vi "Jarvis.vi"() -> ()   [LabVIEW 2019]
uses:
  <vilib>/Utility/miscctls.llb/LVRectTypeDef.ctl
  controls/GlobalExp.vi
  Global.lvlib
  controls/MasterExpControl.ctl
  VIs/Log/GlobalPyConsole.vi
  <vilib>/rvi/interface/nirviOpenFPGA/nirviOpenFPGA.xnode
  <vilib>/rvi/interface/nirviMethod/nirviMethod.xnode
  VIs/GlobalImagingStatus.vi
  controls/ImagingStatusControl.ctl
  controls/xVerticalSlide/XVerticalSlide.xctl
  controls/xHorizontalSlide/XHorizontalSlide.xctl
  VIs/DataFile/DataLock.vi
  VIs/Graphs/GraphsQueue.vi
  controls/xAOMSettings/XAOMsetting.xctl
  <vilib>/rvi/interface/nirviReadWriteControl/nirviReadWriteControl.xnode
  NiFpgaLv.dll
  <vilib>/Utility/error.llb/Error Cluster From Error Code.vi
  <vilib>/rvi/interface/Simulation/niFpgaSimulationCallBeginRW.vi
  <vilib>/rvi/errors/niLvFpgaAdjustHostInterfaceError.vi
  <vilib>/rvi/interface/nirviCloseFPGA/nirviCloseFPGA.xnode
  VIs/Camera/GlobalCamSettings.vi
  controls/AgilentCtrlEnum.ctl
  FPGA_bitfile/Jarvis_FPGATargetMacro_281119TDCLV2017_HUsPPJBlkv4.lvbitx
  <vilib>/FPGAPlugInAG/Dynamic/niLvFpga_ConfigureFifo_Dynamic.vi
  <vilib>/rvi/errors/niLvFpgaMergeErrorWithErrorCode.vi
  <vilib>/FPGAPlugInAG/Dynamic/niLvFpga_Close_Dynamic.vi
  <vilib>/Utility/file.llb/Write Delimited Spreadsheet (DBL).vi
  <vilib>/FPGAPlugInAG/Dynamic/niLvFpga_ReadFifo_Dynamic.vi
  <vilib>/Utility/file.llb/Write Delimited Spreadsheet (I64).vi
  <vilib>/FPGAPlugInAG/PXI-7842R/niLvFpga_Open_PXI-7842R.vi
  <vilib>/rvi/interface/common/dynamic/niFpgaDynamicAddResources.vi
  <vilib>/Utility/file.llb/Read Delimited Spreadsheet (DBL).vi
  VIs/Qalibrate/exp_status.vi
  VIs/PulseCompiler/CompilerSettings.ctl
  controls/ConnectionStatus.ctl
  controls/FilePaths.ctl
  VIs/Mathematica/MathematicaSettingsCtl.ctl
  VIs/Meta/QueueControl.ctl
  controls/ReadoutSettings.ctl
  VIs/Camera/CameraCoordsControl.ctl
  controls/xTextCode/XTextCode.xctl
  controls/PltImageControl.ctl
  controls/FluoSettings.ctl
  controls/CompCoilControl.ctl
  VIs/RSNRPZ/RSNRPZcontrol.ctl
  controls/ControllerSettings.ctl
  controls/PowerStableSettings.ctl
  <vilib>/userDefined/High Color/nirio_resource_hc.ctl
  controls/AWGchannelcontrol.ctl
  controls/AWGpulse.ctl
  VIs/Shutters/XControl/XControlShutter.xctl
panel:
  out "output 2":i32
  out "time string":string
  in  "dummy cluster":T1
  in  "935 cluster":T1 {"wavelength" format="%_8g"}
  in  "399 cluster":T1 {"wavelength" format="%_8g"}
  in  "739 cluster":T1 {"wavelength" format="%_8g"}
  in  "MasterTabCtl":T2(tab)
  in  "ExperimentTab":enum32{"Control", "Meta Queue", "Settings"}(tab)
  out "runs slider":dbl(slide) scale=0.0..1.0
  out "ExpNumIndicator":string="Experiment # : 000"
  in  "Main/Meta":bool
  in  "RunExp":bool
  out "ExpLog":string="28/02/19 Experiment Logbook:\n000: Frequency scan plus1\n001: Two ion state detection\nError: Interrupted during run 23, lost probe lock."
  out "steps slider":dbl(slide) scale=0.0..1.0
  in  "Pause/Stop":cluster{"Exp Stop":bool, "Pause":bool}
  in  "QueueControl":T3
  in  "LoadExpLog":bool
  in  "SaveExpLog":bool
  in  "ControllerSettings":T4={"Aux Sequence"=FALSE, "Camera"=FALSE, "Recrystallize"=TRUE, "Raw graph"=TRUE, "Mean graph"=TRUE, "Calculate probs"=TRUE, "Find fit"=TRUE, "ReX Time [s] :"=20.0, "Lock Voltage :"=220.0, "Line trig "=FALSE, "Check Fluo"=FALSE, "Pre Sequence"=FALSE}
  out "Aux graph":cluster{dbl, dbl}(graph)
  out "Raw graph":dbl[][](graph)
  out "Mean graph":dbl[][](graph)
  out "Proc. graph":dbl[][](graph)
  out "PltPic":picture
  in  "MathImageCtl":T5={"Date:"="", "Exp Num:"="", "Reload"=FALSE, "Auto update : "=TRUE, "String"=""}
  out "String 3":string="Meta  :"
  in  "MetaPush":bool
  in  "MetaSave":bool
  in  "MetaLoad":bool
  out "Python Console":string
  in  "Param Cfg Path":path=path "C:/Users/cv222/Documents/Jarvis/config/parameter_config.ini"
  in  "Param Cfg add":bool
  in  "Param Cfg Save":bool
  in  "Param Cfg Load":bool
  in  "ConfigHeader":string(combo)
  out "String 2":string="Aux  :"
  out "String":string="Main : "
  in  "AuxCompile":bool
  in  "AuxSave":bool
  in  "AuxLoad":bool
  in  "MainCompile":bool
  in  "MainSave":bool
  in  "MainLoad":bool
  in  "ScriptsTab":T6(tab)
  in  "MainPulsecode":string(xcontrol)
  in  "AuxPulseCode":string(xcontrol)
  in  "MetaPulseCode":string(xcontrol)
  in  "ParamCfgList":string[][](array[string])
  in  "NumIonsProcProbs":bool
  in  "Step Number :":dbl
  in  "AverageCamera":bool
  in  "DisplayImage":bool
  in  "InfoTxtList":string[](array[string])
  in  "Analyze Probs":bool
  in  "Find Probabilites":bool
  in  "Process Statedet":bool
  out "Prob graph":dbl[][](graph)
  out "PostProcImg":picture
  out "Console Out":string
  out "Python Error Out":string
  in  "TreeFolderPath":path=path "C:/Users/labadmin/Documents/Jarvis/data" caption="Base Path"
  in  "DataTree":string(tree)
  out "PostProcCamImg":dbl[][](graph)
  in  "LoadPulseSeq":bool
  in  "Pulse Sequence Tab":T7(tab)
  in  "AuxPulseSeq":T8(array[cluster])
  in  "MainPulseSeq":T8(array[cluster])
  out "RF sequence array":T9[](array[typedef])
  out "MW sequence array":T9[](array[typedef]) {"Channel Array"."phase det" format="%#_10g"; "Channel Array"."amp det" format="%#_10g"; "Channel Array"."freq" format="%#_10g"}
  out "AWGgraph":dbl(graph)
  in  "UpdateAWGSeqGraph":bool
  out "pulseseq parameter config":string
  out "Fluorescence :":dbl
  in  "Shutdown Status :":string
  in  "DisconnectCamera":bool
  in  "CamFluo selector":string(combo)="Large View"
  in  "Large cam coords":T11={"Top :"=450.0, "Bottom :"=280.0, "Left :"=340.0, "Right :"=530.0} caption="Camera Coordinates"
  in  "CamXSlide":cluster{"low":i16, "high":i16}(xcontrol)={"low"=318, "high"=527}
  in  "CamYSlider":cluster{"low":i16, "high":i16}(xcontrol)={"low"=194, "high"=343}
  in  "ion coords":T11={"Top :"=681.0, "Bottom :"=691.0, "Left :"=393.0, "Right :"=406.0}
  out "Big Camera":dbl[][](graph)
  out "CamFluoChart":cluster{"Frequency Chart":u32, "mean":dbl}(graph)
  out "Left ion graph":dbl[][](graph)
  out "Rolling average :":dbl format="%_4g"
  in  "Agilient visa":string="TCPIP0::192.168.1.203::inst0::INSTR" caption="Agilient VSG Resource Name :"
  in  "RSNPRZsettings":T12={"Average Counts :"=1.0, "Correction Freq [MHz] :"=50.0, "Integration Time [ms] : "=0.1, "P :"=0.0, "I :"=0.0, "D :"=0.0, "Power setpoint :"=0.0, "PID on :"=FALSE, "Voltage :"=0.0, "Reset :"=FALSE, "Agilient Power Level [dBm] :"=0.0} caption="RSNPRZ Settings :" {"Agilient Power Level [dBm] :" format="%_4g"; "Voltage :" format="%_5g"; "Power setpoint :" format="%_4g"; "D :" format="%_4g"; "I :" format="%_4g"; "P :" format="%_4g"; "Integration Time [ms] :" format="%_3g"; "Correction Freq [MHz] :" format="%_4g"}
  in  "rsnrpz rsrc name":string="USB::0x0aad::0x00a7::101568" caption="RSNRPZ Resource Name :"
  out "RSNPRZgraph":dbl(graph)
  out "AWGContMSG":string caption="AWG Instrument Response"
  in  "UpdateAWGGraph":bool
  out "Wave Form preview":cluster{"X":dbl, "Y":dbl}[](graph)
  in  "LoadWaveforms":bool
  in  "SaveWaveformsToFile":bool
  in  "SendWaveformToAWG":bool
  in  "Tab Control 2":enum32{"Microwave", "RF"}(tab)
  in  "ArbitraryWaveListTitle":string[][](array[string])=[["Frequency [MHz]", "Amplitude [mV]", "Phase"]] caption="AWGListTitle"
  in  "ArbitraryWaveListMW":dbl[][](array[numeric])=[[100014.0, 200.0, 0.0], [105000.0, 100.0, 0.0], [95000.0, 100.0, 0.0]] caption="Arbitrary Waveform List"
  in  "ArbitraryWaveListRF":dbl[][](array[numeric])=[[100014.0, 200.0, 0.0], [105000.0, 100.0, 0.0], [95000.0, 100.0, 0.0]] caption="Arbitrary Waveform List"
  in  "ArbitraryWaveListTitle 2":string[][](array[string])=[["Frequency [MHz]", "Amplitude [mV]", "Phase"]] caption="AWGListTitle"
  in  "AO cluster":T13
  in  "DIOcluster":T14
  out "AnalogOutput":T15 {"AI 7" scale=0.0..10.0; "AI 6" scale=0.0..10.0; "AI 5" scale=0.0..10.0; "AI 4" scale=0.0..10.0; "AI 3" scale=0.0..10.0; "AI 2" scale=0.0..10.0; "AI 1" scale=0.0..10.0; "AI 0" scale=0.0..10.0}
  in  "369 unlock notification":bool
  in  "VISA: Pressure":refnum<visa-resource-name>
  in  "Tab control":cluster{"visible":bool, "Tab name":string}[](array[cluster])=[{"visible"=TRUE, "Tab name"="Experiment Controller"}, {"visible"=TRUE, "Tab name"="Pulse Programming"}, {"visible"=TRUE, "Tab name"="Pulse Sequence"}, {"visible"=FALSE, "Tab name"="DDS Boards"}, {"visible"=FALSE, "Tab name"="Calypso"}, {"visible"=TRUE, "Tab name"="Digital/Analog"}, {"visible"=FALSE, "Tab name"="Cryo DC"}, {"visible"=FALSE, "Tab name"="Cryo Control"}, {"visible"=TRUE, "Tab name"="Beam Blockers"}]
  in  "LoadSession":bool
  in  "SaveSession":bool
  in  "Mathematica Settings":T16
  in  "Connection Status":T17={"Newton"=TRUE, "Camera"=TRUE, "Atlas"=TRUE, "Pressure"=TRUE, "AWG"=TRUE, "DDS A"=TRUE, "DDS B"=TRUE, "DDS C"=TRUE, "DDS D"=TRUE, "rsnrpz"=TRUE}
  out "GlobalLog":string
  in  "Compiler Settings":T18={"Python Path"=path "", "Main File"="scriptmain.py", "Meta File"="scriptmeta.txt", "Aux File"="scriptaux.py", "Pre File"="scriptpre.py"}
  in  "File Paths":T19={"Local Save Path"=path "C:/Users/cv222/Documents/Jarvis/data", "Newton Save Path"=path "Z:/#Projects/Entanglement/data", "File Name"="test", "LocalSave"=TRUE}
  out "rsnrpz VISA session":refnum<visa-resource-name> caption="VISA resource name"
  in  "FPGA address":T20="PXI1Slot2" caption="RIO Device"
  in  "camera debug":bool
  in  "Stop":bool
  out "Waveform Chart":i32[](graph)
  out "Current iteration":u32
  in  "N measurements":dbl
  in  "Run TDC":bool
  out "FPGAerr":bool=TRUE
  out "Laser status":bool[](array[boolean])
  out "AtlatsStat":string[](array[string])
  in  "Readout Settings":T21={"1ion t'hold (>=)"=3, "2 ion levels?"=FALSE, "2ion t'hold (>=)"=0, "Cam Thresholds"=[4650, 4650], "Region size"=0, "Ion 1 centre x"=3, "Ion 1 centre y"=3, "Ion 2 centre x"=3, "Ion 2 centre y"=3}
  in  "SessionWindowShow":bool
  in  "Global status":enum16{"Idle", "Pulse", "Calypso"}(ring)=enum."Calypso"
  in  "ImagingStatus":enum16{"PMT", "Camera", "Idle"}(ring)=enum."Idle"
  out "Running VIs ref":refnum<vi>[](array[refnum])
  out "queue out":refnum<queue>
  in  "QueueChanged":bool=TRUE
  in  "Stop button":bool
  out "Title":string="Jarvis - IQT Sussex"
  out "Pressure":dbl
  out "Photodiode":dbl
  in  "Small View Tab":enum32{"PMT", "Camera"}(tab)
  out "PMT chart":i32(graph)
  out "Small Camera":dbl[][](graph)
  in  "ExtraTabControl":T22(tab)
  in  "AOMsetting":T23(xcontrol)
  in  "FluoSettings":T24={"Lock Fluorescence"=FALSE, "Aux runs : "=1, "Loop on test :"=FALSE, "Loop frequency : "=FALSE, "Frequency Min"=110.0, "Frequency Max"=130.0, "PMT"={"Lock point : "=68.0, "dF/dFl"=-0.04, "Unlock min"=66.0, "Unlock max"=70.0, "Loop min"=50.0, "Loop max"=160.0}, "Camera"={"Lock point : "=68.0, "dF/dFl"=-0.04, "Unlock min"=66.0, "Unlock max"=70.0, "Loop min"=50.0, "Loop max"=160.0}} {"Camera"."dF/dFl" format="%.2f"; "PMT"."dF/dFl" format="%.2f"}
  in  "CompCoilSettings":T25
  in  "PowerStableSettings":T26={"Lock Power"=TRUE, "Number measurements"=10, "Min AWG Power [dBm] :"=0.0, "Max AWG Power [dBm] :"=1.0, "Min Power Difference [dBm] : "=-1.0, "Max Power Difference [dBm] :"=1.0, "Agilient visa "="TCPIP0::192.168.1.203::inst0::INSTR"}
  in  "XControlShutter":dbl(xcontrol)
  # "Queue :"
  # "AWG trig"
  # "Cam trig"
  # "UWAVE"
  # "countA"
  # "countC"
  # "countD"
  # "countB"
  # "MW5"
  # "AOM"
  # "MW1"
  # "MW2"
  # "MW3"
  # "MW4"
  # "MW6"
  # "MW7"
  # "MW8"
  # "EOM"
  # "DIO9"
  # "trig1"
  # "AO1"
  # "AO2"
  # "AO3"
  # "AO4"
  # "RF1"
  # "RF2"
  # "RF3"
  # "RF5"
  # "RF6"
  # "XM"
  # "RF4"
  # "XR"
  # "Main Sequence"
  # "Auxiliary Sequence"
  # "Name :"
  # "Timing :"
  # "Detuning :"
  # "Step :"
  # "Frequency :"
  # "Step :"
  # "Amplitude :"
  # "Step :"
  # "Phase  :"
  # "Step :"
  # "Name :"
  # "Timing :"
  # "Detuning :"
  # "Step :"
  # "Frequency :"
  # "Step :"
  # "Amplitude :"
  # "Step :"
  # "Phase  :"
  # "Step :"
  # "AOM"
  # "CAM"
  # "MW7"
  # "MW8"
  # "XM"
  # "RF"
  # "XR"
  # "AOM"
  # "EOM"
  # "MW"
  # "MW1"
  # "MW2"
  # "MW3"
  # "MW4"
  # "MW5"
  # "MW6"
  # "Current lock :"
  # "Unlock if :"
  # "Probability lock :"
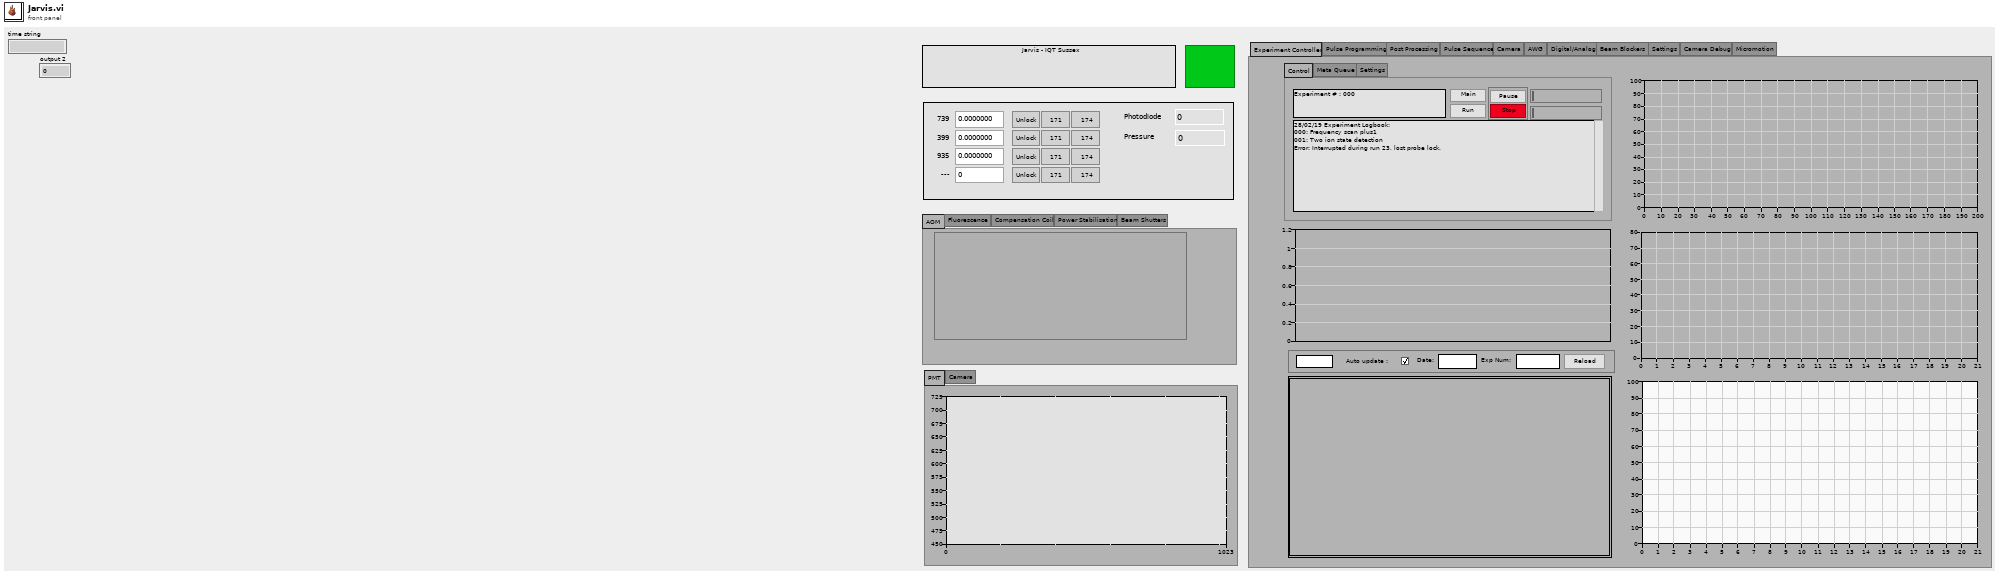
[diagram p1: front panel]
types:
  T1 = cluster{"wavelength":dbl, "unlock":bool, "unlock 2":bool, "unlock 3":bool}
  T2 = enum32{"Experiment Controller", "Pulse Programming", "Post Processing", "Pulse Sequence", "Camera", "AWG", "Calypso", "Digital/Analog", "Beam Blockers", "Cryo Control", "Cryo DC", "Settings", "Camera Debug", "Micromotion", "Debug", "Misc"}
  T3 = typedef "QueueControl.ctl" = cluster{"QueueFromServer":i32, "First Queue":string, "Add To Queue:":string, "Up":bool, "Down":bool, "Del":bool, "Front":bool, "Back":bool, "Next":bool, "Combo Box":string}
  T4 = typedef "ControllerSettings.ctl" = cluster{"Aux Sequence":bool, "Camera":bool, "Recrystallize":bool, "Raw graph":bool, "Mean graph":bool, "Calculate probs":bool, "Find fit":bool, "ReX Time [s] :":dbl, "Lock Voltage :":dbl, "Line trig ":bool, "Check Fluo":bool, "Pre Sequence":bool}
  T5 = typedef "PltImageControl.ctl" = cluster{"Date:":string, "Exp Num:":string, "Reload":bool, "Auto update : ":bool, "String":string}
  T6 = enum32{"Main Script", "Aux Script", "Meta Script"}
  T7 = enum32{"FPGA Sequence", "AWG Sequence", "Parameter Config"}
  T8 = cluster{"String":string, "Numeric":dbl, "Boolean":bool, "Numeric 2":dbl, "Numeric 3":dbl, "Boolean 2":bool, "Boolean 3":bool, "Boolean 4":bool, "Boolean 5":bool, "Boolean 6":bool, "Boolean 7":bool, "Boolean 8":bool, "Boolean 9":bool, "Boolean 10":bool, "Boolean 11":bool, "Boolean 12":bool, "Boolean 13":bool, "Boolean 14":bool, "Boolean 15":bool, "Boolean 16":bool, "Boolean 17":bool, "Boolean 18":bool, "Boolean 19":bool, "Boolean 20":bool, "Boolean 21":bool, "Boolean 22":bool, "Boolean 23":bool, "Boolean 24":bool, "Boolean 25":bool, "Boolean 26":bool, "Boolean 27":bool, "Boolean 28":bool, "Boolean 29":bool, "Boolean 30":bool, "Boolean 31":bool, "Boolean 32":bool, "Boolean 33":bool, "Boolean 34":bool, "Boolean 35":bool, "Boolean 36":bool, "Boolean 37":bool, "Boolean 38":bool, "Boolean 39":bool, "Boolean 40":bool, "Boolean 41":bool, "Boolean 42":bool, "Boolean 43":bool, "Boolean 44":bool, "Boolean 45":bool, "Boolean 46":bool, "Boolean 47":bool, "Boolean 48":bool, "Boolean 49":bool, "Boolean 50":bool, "Boolean 51":bool, "Boolean 52":bool, "Boolean 53":bool, "Boolean 54":bool}[]
  T9 = typedef "AWGpulse.ctl" = cluster{"Name":string, "time det":dbl, "time step":dbl, "Channel Array":T10[]}
  T10 = typedef "AWGchannelcontrol.ctl" = cluster{"freq\n":dbl, "freq step":dbl, "amp det":dbl, "amp step":dbl, "phase det":dbl, "phase step":dbl}
  T11 = typedef "CameraCoordsControl.ctl" = cluster{"Top :":dbl, "Bottom :":dbl, "Left :":dbl, "Right :":dbl}
  T12 = typedef "RSNRPZcontrol.ctl" = cluster{"Average Counts :":dbl, "Correction Freq [MHz] :":dbl, "Integration Time [ms] : ":dbl, "P :":dbl, "I :":dbl, "D :":dbl, "Power setpoint :":dbl, "PID on :":bool, "Voltage :":dbl, "Reset :":bool, "Agilient Power Level [dBm] :":dbl}
  T13 = cluster{"AO 0":dbl, "AO 1":dbl, "AO 2":dbl, "AO 3":dbl, "AO 4":dbl, "AO 5":dbl, "AO 6":dbl, "AO 7":dbl}
  T14 = cluster{"DIO 0":bool, "DIO 1":bool, "DIO 2":bool, "DIO 3":bool, "DIO 4":bool, "DIO 5":bool, "DIO 6":bool, "DIO 7":bool, "DIO 8":bool, "DIO 9":bool, "DIO 10":bool, "DIO 11":bool, "DIO 12":bool, "DIO 13":bool, "DIO 14":bool, "DIO 15":bool, "DIO 16":bool, "DIO 17":bool, "DIO 18":bool, "DIO 19":bool, "DIO 20":bool, "DIO 21":bool, "DIO 22":bool, "DIO 23":bool, "DIO 24":bool, "DIO 25":bool, "DIO 26":bool, "DIO 27":bool, "DIO 28":bool, "DIO 29":bool, "DIO 30":bool, "DIO 31":bool, "DIO 32":bool, "DIO 33":bool, "DIO 34":bool, "DIO 35":bool, "DIO 36":bool, "DIO 37":bool, "DIO 38":bool, "DIO 39":bool}
  T15 = cluster{"AI 0":dbl, "AI 1":dbl, "AI 2":dbl, "AI 3":dbl, "AI 4":dbl, "AI 5":dbl, "AI 6":dbl, "AI 7":dbl}
  T16 = typedef "MathematicaSettingsCtl.ctl" = cluster{"Mathematica Dir":path, "Scripts Dir":path}
  T17 = typedef "ConnectionStatus.ctl" = cluster{"Newton":bool, "Camera":bool, "Atlas":bool, "Pressure":bool, "AWG":bool, "DDS A":bool, "DDS B":bool, "DDS C":bool, "DDS D":bool, "rsnrpz":bool}
  T18 = typedef "CompilerSettings.ctl" = cluster{"Python Path":path, "Main File":string, "Meta File":string, "Aux File":string, "Pre File":string}
  T19 = typedef "FilePaths.ctl" = cluster{"Local Save Path":path, "Newton Save Path":path, "File Name":string, "LocalSave":bool}
  T20 = typedef "nirio_resource_hc.ctl" = tag
  T21 = typedef "ReadoutSettings.ctl" = cluster{"1ion t'hold (>=)":u32, "2 ion levels?":bool, "2ion t'hold (>=)":u32, "Cam Thresholds":u32[], "Region size":i32, "Ion 1 centre x":i32, "Ion 1 centre y":i32, "Ion 2 centre x":i32, "Ion 2 centre y":i32}
  T22 = enum32{"AOM", "Fluorescence", "Compensation Coil", "Power Stabilisation", "Beam Shutters"}
  T23 = cluster{"HighPowerNum":dbl, "LowPowerNum":dbl, "PIDnum":dbl, "DeltaFreq":dbl, "BaseFreq":dbl, "AOMout":dbl, "ButtonSelected":enum16{"PID", "Low", "High"}, "AO3":bool}
  T24 = typedef "FluoSettings.ctl" = cluster{"Lock Fluorescence":bool, "Aux runs : ":i32, "Loop on test :":bool, "Loop frequency : ":bool, "Frequency Min":dbl, "Frequency Max":dbl, "PMT":cluster{"Lock point : ":dbl, "dF/dFl":dbl, "Unlock min":dbl, "Unlock max":dbl, "Loop min":dbl, "Loop max":dbl}, "Camera":cluster{"Lock point : ":dbl, "dF/dFl":dbl, "Unlock min":dbl, "Unlock max":dbl, "Loop min":dbl, "Loop max":dbl}}
  T25 = typedef "CompCoilControl.ctl" = cluster{"Min [mA]":dbl, "Max [mA]":dbl, "Apply lock :":bool, "Unlock min":dbl, "Unlock max":dbl, "Loop current :":bool, "Reset if out of range :":bool, "Aux runs :":i32, "dI [mA] :":dbl, "Prob lock min ":dbl, "Prob lock max":dbl, "Current [mA]":dbl}
  T26 = typedef "PowerStableSettings.ctl" = cluster{"Lock Power":bool, "Number measurements":i32, "Min AWG Power [dBm] :":dbl, "Max AWG Power [dBm] :":dbl, "Min Power Difference [dBm] : ":dbl, "Max Power Difference [dBm] :":dbl, "Agilient visa ":string}
  T27 = typedef "ImagingStatusControl.ctl" = enum16{"PMT_large", "Camera_large", "PMT", "Camera", "Idle"}
  T28 = enum8{"Enabled", "Disabled", "Disabled and Grayed Out"}
  T29 = enum16{"Innit", "Stop", "Idle", "MainRunning", "AuxRunning"}
  T30 = enum32{"Page Enabled", "Page Disabled", "Page Disabled & Grayed"}
  T31 = typedef "MasterExpControl.ctl" = cluster{"Main Steps":dbl, "Main Runs":dbl, "ExpStatus":enum16{"Innit", "Stop", "Idle", "MainRunning", "AuxRunning"}, "Main Current Step":dbl, "ExpNum":dbl, "NewData":bool, "date":string, "command":string, "Stop":bool, "Pause":bool, "Mathematica":string, "Main/Meta":bool, "UpdateMath":bool, "Camera":bool, "MetaExpOver":bool, "NextMetaExp":bool}
  T32 = typedef "LVRectTypeDef.ctl" = cluster{"Left":i16, "Top":i16, "Right":i16, "Bottom":i16}
  T33 = enum16{"del", "update", "down", "up", "bot", "top"}
  T34 = typedef "AgilentCtrlEnum.ctl" = enum16{"WRITE_POW", "READ_POW"}
  T35 = cluster{"Wavelengths[0]":dbl, "Wavelengths[1]":dbl, "Wavelengths[2]":dbl, "Wavelengths[3]":dbl, "Wavelengths[4]":dbl, "Wavelengths[5]":dbl, "Wavelengths[6]":dbl, "Wavelengths[7]":dbl, "Wavelengths[8]":dbl}
  T36 = typedef "SinglePulse.ctl" = cluster{"enabled":bool, "string":string, "time":dbl, "step":dbl, "dio":dbl, "count":dbl, "trigger":dbl, "AO":dbl}
  T37 = cluster{"Pulse name":string, "Pulse number":i32, "Enabled?":bool, "Time":dbl, "Step":dbl, "Pulse 0":bool, "Pulse 1":bool, "Pulse 2":bool, "Pulse 3":bool, "Pulse 4":bool, "Pulse 5":bool, "Pulse 6":bool, "Pulse 7":bool, "Pulse 8":bool, "Pulse 9":bool, "Pulse 10":bool, "Pulse 11":bool, "Pulse 12":bool, "Pulse 13":bool, "Pulse 14":bool, "Pulse 15":bool, "Pulse 16":bool, "Pulse 17":bool, "Pulse 18":bool, "Pulse 19":bool, "Pulse 20":bool, "Pulse 21":bool, "Pulse 22":bool, "Pulse 23":bool, "Pulse 24":bool, "Pulse 25":bool, "Pulse 26":bool, "Pulse 27":bool, "Pulse 28":bool, "Pulse 29":bool, "Pulse 30":bool, "Pulse 31":bool, "Pulse 32":bool, "Pulse 33":bool, "Pulse 34":bool, "Pulse 35":bool, "Pulse 36":bool, "Pulse 37":bool, "Pulse 38":bool, "Pulse 39":bool, "Count 0":bool, "Count 1":bool, "Count 2":bool, "Count 3":bool, "Count 4":bool, "Count 5":bool, "Count 6":bool, "Count 7":bool, "AO 0":bool, "AO 1":bool, "AO 2":bool, "AO 3":bool, "Trigger 0":bool}[]
  T38 = typedef "CameraSettings.ctl" = cluster{"EM Gain :":dbl, "Pre Amp Gain :":dbl, "VS Speed [Index] :":dbl, "VS Amplitude :":dbl, "Exposure Time [s] :":dbl, "Temperature :":dbl, "HS Speed [s]":dbl, "Gain > 300 :":bool}
  T39 = cluster{"number: 0 to 1":dbl, "number: 0 to 1":dbl}
  T40 = cluster{"steps slider":refnum<vi>, "runs slider":refnum<vi>}
  T41 = cluster{"CompCoilSettings":refnum<vi>, "FluoSettings":refnum<vi>, "AOMsetting":refnum<vi>, "PowerStableSettings":refnum<vi>}
  T42 = cluster{"StepsSlider":refnum<vi>, "runs slider":refnum<vi>}
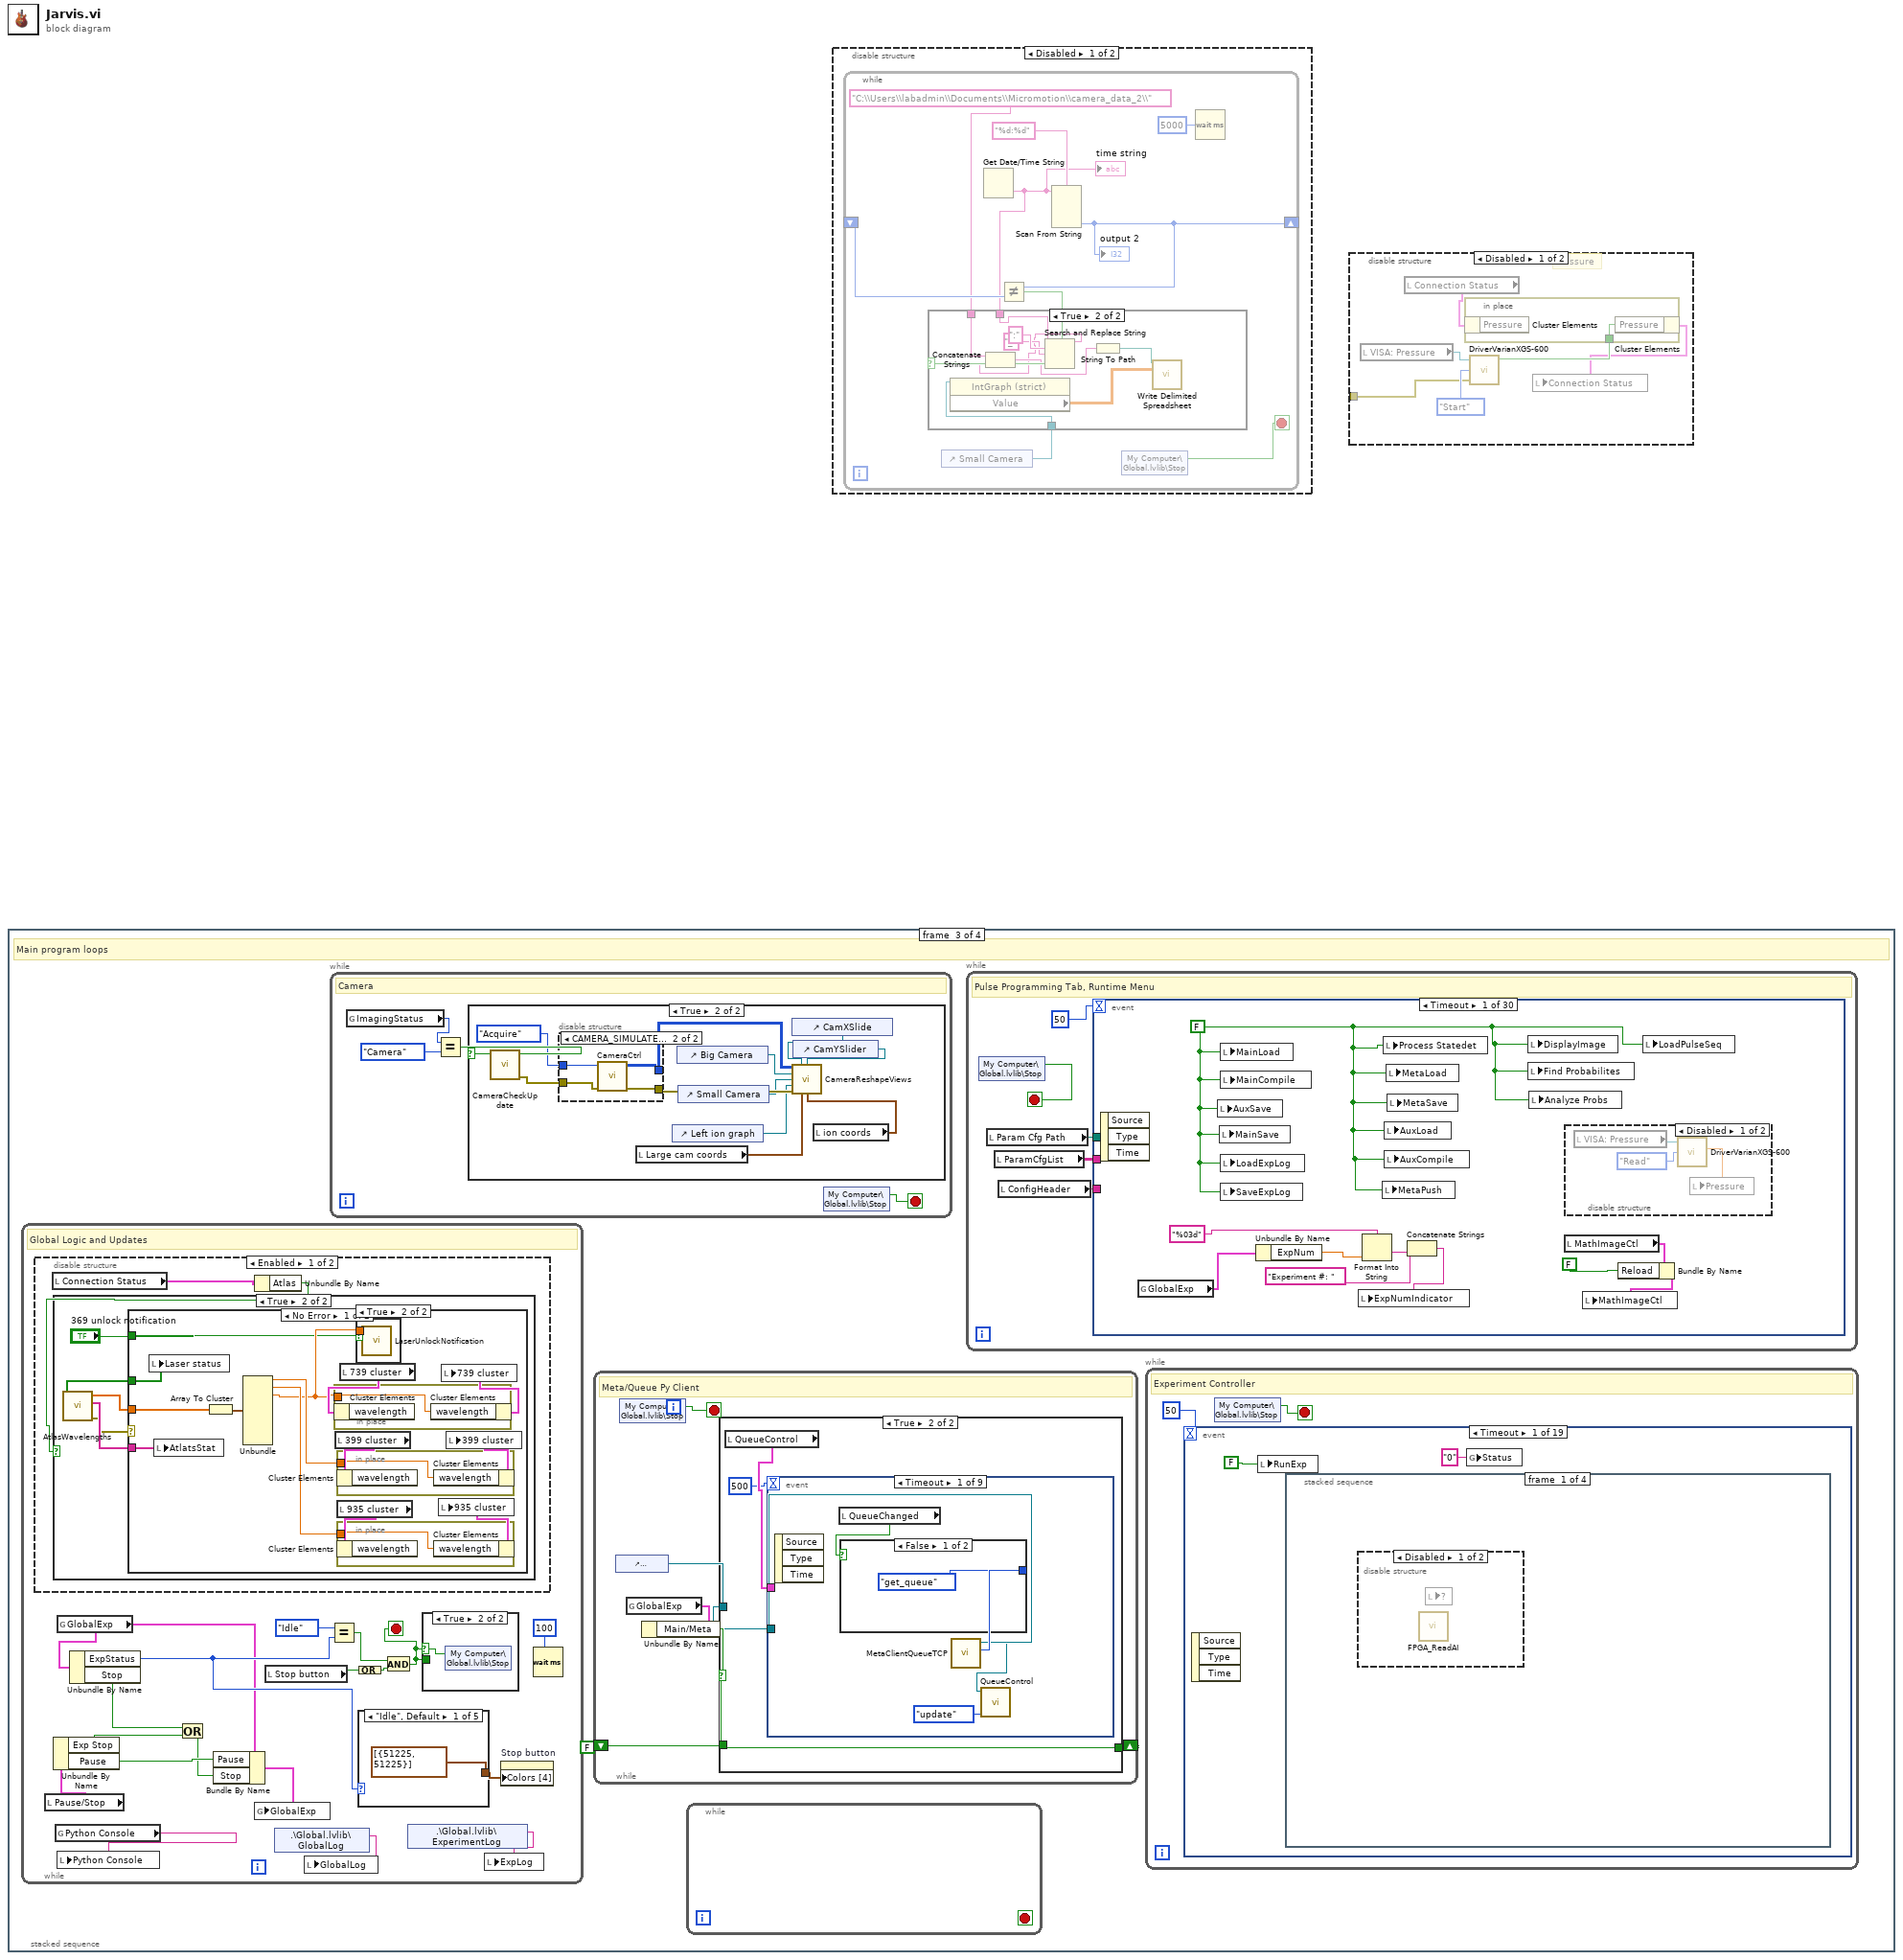
[diagram p0: block diagram]
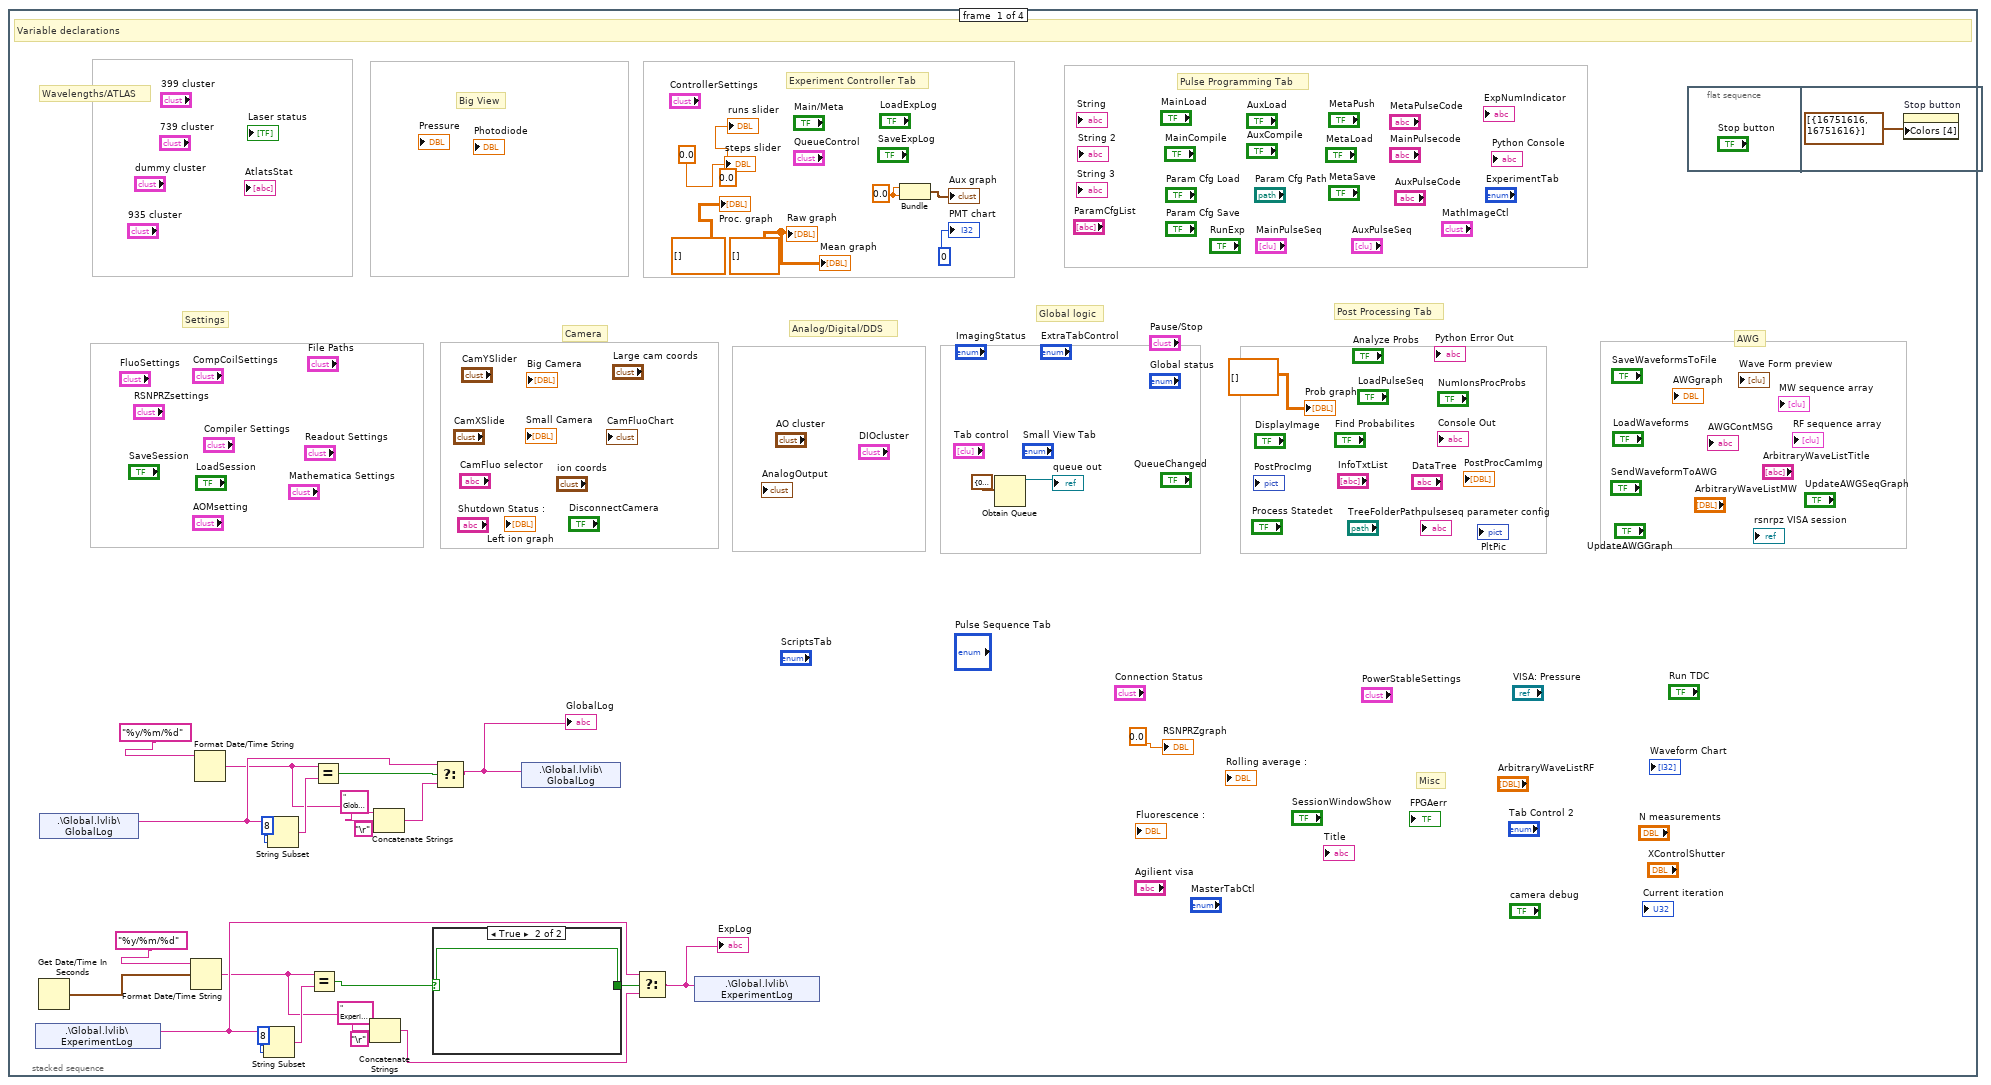
[diagram p5: hidden frame]
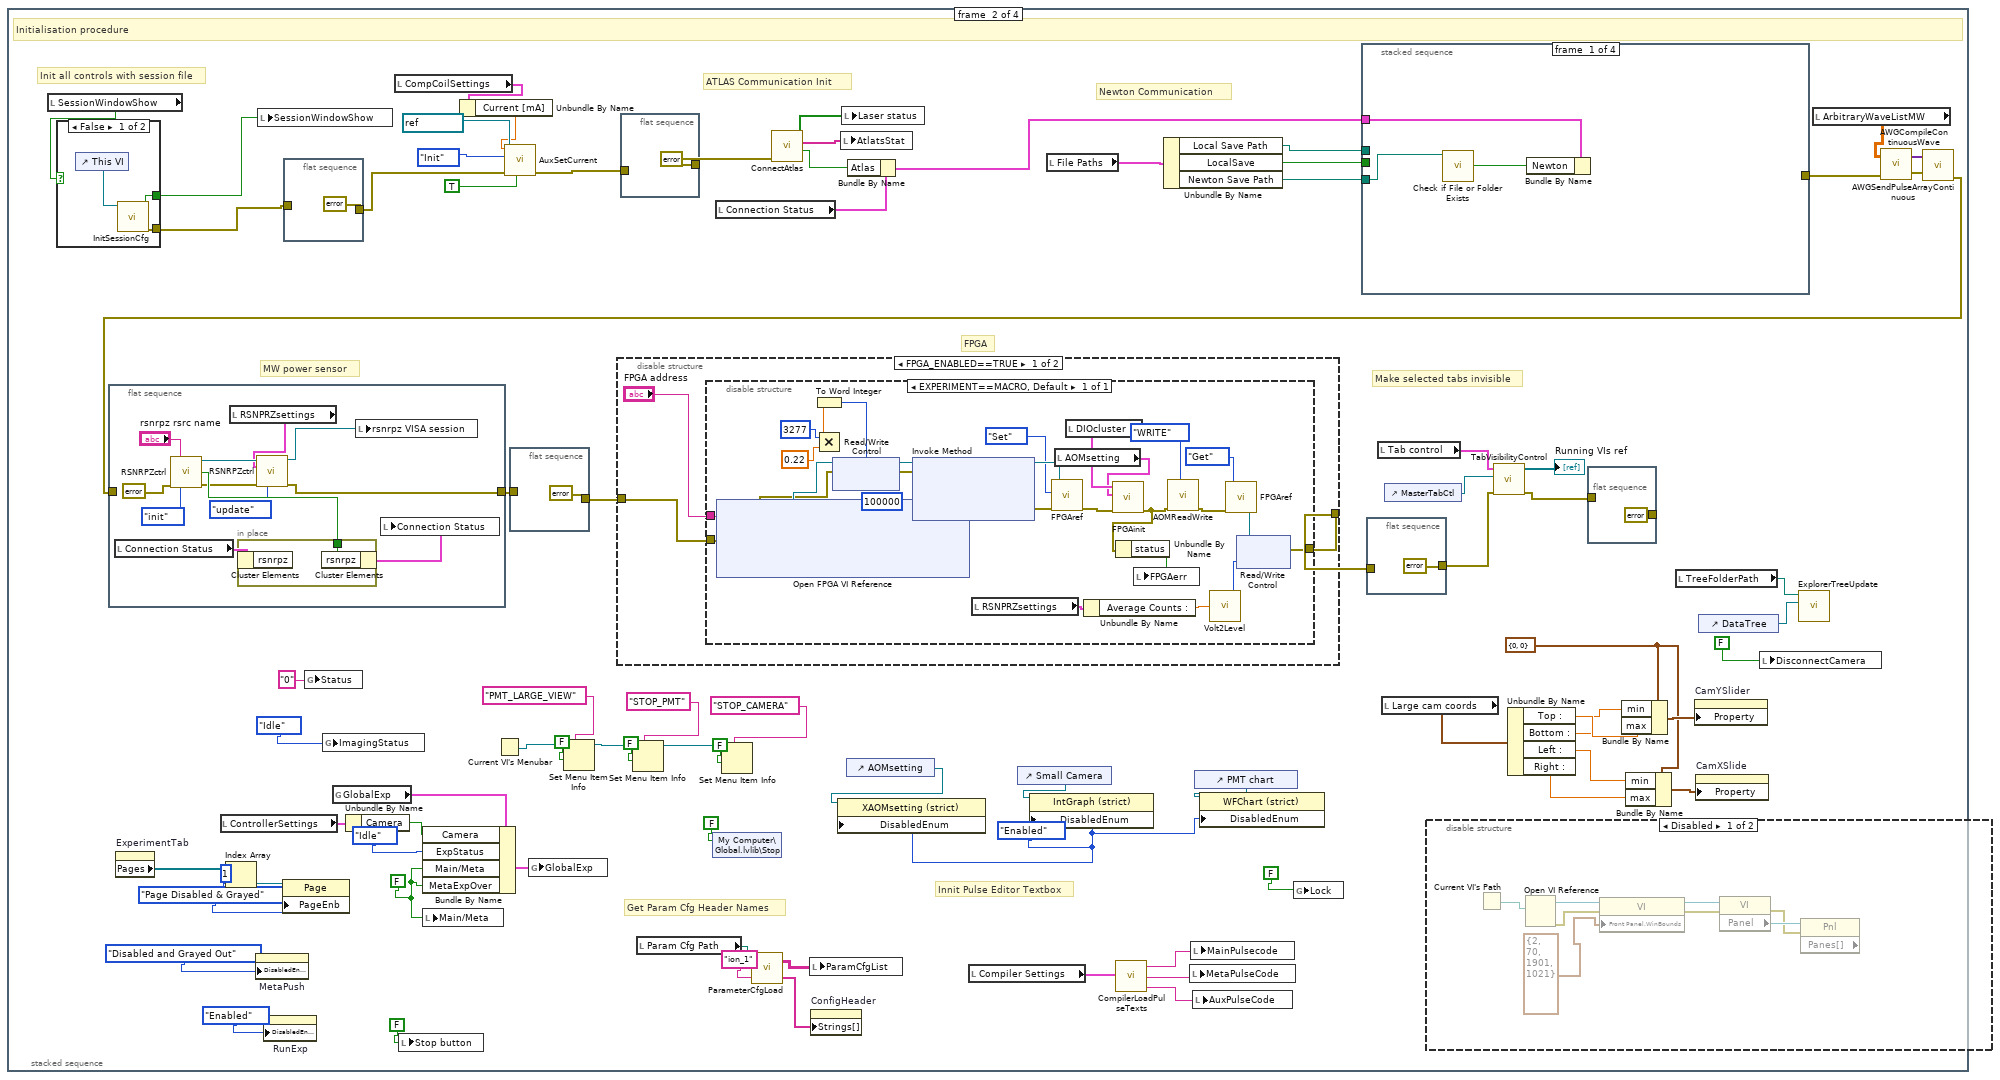
[diagram p7: hidden frame]
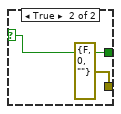
[diagram p9: hidden frame]
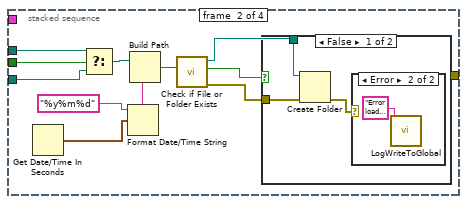
[diagram p10: hidden frame]
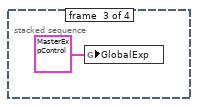
[diagram p13: hidden frame]
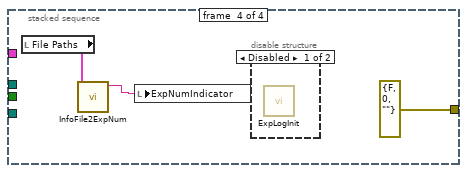
[diagram p14: hidden frame]
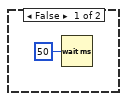
[diagram p17: hidden frame]
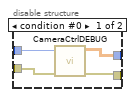
[diagram p18: hidden frame]
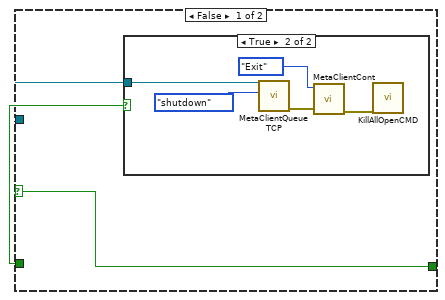
[diagram p19: hidden frame]
diagram:
  n1 = stacked-sequence {
    frame #0 {
      w5 = 0.0
      w23 = dbl[][] []
      # "AWG"
      # "Misc"
      # "Post Processing Tab"
      # "Global logic"
      # "Analog/Digital/DDS"
      # "Settings"
      # "Camera"
      # "Big View"
      # "Experiment Controller Tab"
      # "Pulse Programming Tab"
      # "Wavelengths/ATLAS"
      # "Variable declarations"
      n2 = shared-variable ".\\Global.lvlib\\ExperimentLog"() -> (w30:string)  [unwired: 1 in, 1 out]
      n3 = Get Date/Time In Seconds() -> (seconds since 1Jan1904=w31:timestamp)
      n4 = shared-variable ".\\Global.lvlib\\GlobalLog"() -> (w20:string)  [unwired: 1 in, 1 out]
      n5 = Format Date/Time String(time format string (%c)="%y/%m/%d", seconds (now)=w31) -> (date/time string=w24:string)  [unwired: 1 in]
      n6 = Format Date/Time String(time format string (%c)="%y/%m/%d") -> (date/time string=w15:string)  [unwired: 2 in]
      n7 = String Subset(string=w30, length (rest)=8 ("length (rest)")) -> (substring=w26:string)  [unwired: 1 in]
      n8 = String Subset(string=w20, length (rest)=8 ("length (rest)")) -> (substring=w16:string)  [unwired: 1 in]
      n9 = Equal?(x=w24, y=w26) -> (x = y?=w13:bool)
      n10 = Equal?(x=w15, y=w16) -> (x = y?=w14:bool)
      n11 = Concatenate Strings(w24, " Experiment Logbook:" ("string"), "\r") -> (w27:string)
      n12 = Concatenate Strings(w15, " Global Log:" ("string"), "\r") -> (w17:string)
      n13 = case shown="True" w13 {
        selector: w13 -> [w35 w36]
        tunnel: [w35 w36] -> w12
        frame False {
        }
        frame True {
        }
      }
      n14 = Select(t=w20, s=w14, f=w17) -> (s? t:f=w11:string)
      "GlobalLog" <- w11
      n15 = shared-variable ".\\Global.lvlib\\GlobalLog"(w11) -> ()  [unwired: 1 in, 1 out]
      n16 = Select(t=w30, s=w12, f=w27) -> (s? t:f=w25:string)
      "ExpLog" <- w25
      n17 = shared-variable ".\\Global.lvlib\\ExperimentLog"(w25) -> ()  [unwired: 1 in, 1 out]
      n18 = Bundle(w5, w5) -> (→"Aux graph":cluster{dbl, dbl})  [unwired: 1 in]
      n19 = Obtain Queue(element data type=cluster{dbl, dbl} {0.0, 0.0}) -> (queue out=→"queue out":refnum<queue>)  [unwired: 4 in, 2 out]
      n20 = flat-sequence {
        frame #0 {
        }
        frame #1 {
          n21 = property on="Stop button" class="Bool (strict)"("Colors [4]"=cluster{u32, u32}[] [{16751616, 16751616}]) -> ()  [unwired: 2 in, 2 out]
        }
      }
      "Proc. graph" <- dbl[][] []
      "Mean graph" <- w23
      "Raw graph" <- w23
      "runs slider" <- 0.0 ("runs slider")
      "steps slider" <- 0.0 ("steps slider")
      "PMT chart" <- 0
      "Prob graph" <- dbl[][] []
      "RSNPRZgraph" <- 0.0
    }
    frame #1 {
      w77 = cluster{"min":i16, "max":i16} {"min"=0, "max"=0} ("SlideBounds")
      w60 = T28."Enabled" ("Disabled")
      w51 = FALSE ("Main/Meta")
      # "MW power sensor"
      # "FPGA"
      # "Init all controls with session file"
      # "Make selected tabs invisible"
      # "Innit Pulse Editor Textbox"
      # "Get Param Cfg Header Names"
      # "Newton Communication"
      # "ATLAS Communication Init"
      # "Initialisation procedure"
      n22 = local read "SessionWindowShow"() -> (w99:bool)
      n23 = case shown="False" w99 {
        selector: w99 -> [_ w172]
        tunnel: [w171 errorcluster {"status"=FALSE, "code"=0, "source"=""} ("error out")] -> w48
        tunnel: [w169 w172] -> w98
        frame False {
          n24 = control-ref of="This VI"() -> (w170:refnum<vi>)
          n25 = call "InitSessionCfg.vi"("This VI"=w170) -> ("error out"=w171:errorcluster, "Showagian 2"=w169:bool)  [unwired: 9 in]
        }
        frame True {
        }
      }
      n26 = flat-sequence {
        tunnel: w52 -> [_]
        tunnel: [w159] -> w59
        frame #0 {
          n27 = local read "Connection Status"() -> (w165:T17)
          n28 = call "RSNRPZctrl.vi"("Resource Name (USB::0x0aad::0x000b::100000)"="rsnrpz rsrc name", "error in (no error)"=errorcluster {"status"=FALSE, "code"=0, "source"=""}, "action"=enum16{"close", "update", "read", "init"}."init") -> ("dup VISA session out"=w162:refnum<visa-resource-name>, "connection status"=w164:bool, "error out"=w161:errorcluster)  [unwired: 9 in, 1 out]
          n29 = local read "RSNPRZsettings"() -> (w156:T12)
          n30 = in-place {
            in-place-border: w164 -> [w168]
            n31 = in-place-cluster #1(w165) -> ()  [unwired: 1 out]
            n32 = in-place-cluster #1("rsnrpz"=w168) -> (w163:T17)
          }
          n33 = call "RSNRPZctrl.vi"("VISA session in"=w162, "RSNPRZsettings"=w156, "error in (no error)"=w161, "action"=enum16{"close", "update", "read", "init"}."update") -> ("dup VISA session out"=w160:refnum<visa-resource-name>, "error out"=w159:errorcluster)  [unwired: 8 in, 2 out]
          n34 = local write "rsnrpz VISA session"(w160) -> ()
          n35 = local write "Connection Status"(w163) -> ()
        }
      }
      n36 = property on="ExperimentTab" class="TabCtl (strict)"() -> ("Pages"=w104:refnum<vi>[])  [unwired: 2 in, 2 out]
      n37 = local read "ControllerSettings"() -> (w68:T4)
      n38 = Index Array(array=w104, index=1) -> (element=w103:refnum<vi>)
      n39 = property on="MetaPush" class="Bool (strict)"("DisabledEnum"=T28."Disabled and Grayed Out" ("Disabled")) -> ()  [unwired: 2 in, 2 out]
      n40 = local write "SessionWindowShow"(w98) -> ()
      n41 = property on="RunExp" class="Bool (strict)"("DisabledEnum"=T28."Enabled" ("Disabled")) -> ()  [unwired: 2 in, 2 out]
      n42 = property class="Page"(reference=w103, "PageEnb"=T30."Page Disabled & Grayed" ("Page Enabled State")) -> ()  [unwired: 1 in, 2 out]
      n43 = flat-sequence {
        tunnel: [errorcluster {"status"=FALSE, "code"=0, "source"=""} ("error out")] -> w47
        tunnel: w48 -> [_]
        frame #0 {
        }
      }
      n44 = global write "exp_status.vi" "Status"("0" ("Status")) -> ()
      n45 = global write "GlobalImagingStatus.vi" "ImagingStatus"(ImagingStatusControl."Idle" ("ImagingStatus")) -> ()
      n46 = global read "GlobalExp.vi" "GlobalExp"() -> (w108:T31)
      n47 = Unbundle By Name(w68) -> ("Camera"=w67:bool)
      n48 = local read "CompCoilSettings"() -> (w42:T25)
      n49 = local write "Stop button"(FALSE ("Stop button")) -> ()
      n50 = Bundle By Name(cluster=w108, "Camera"=w67, "ExpStatus"=T29."Idle", "Main/Meta"=w51, "MetaExpOver"=w51) -> (w107:T31)
      n51 = local write "Main/Meta"(w51) -> ()
      n52 = Unbundle By Name(w42) -> ("Current [mA]"=w41:dbl)
      n53 = Current VI's Menubar() -> (w87:refnum<k9>)
      n54 = call "AuxSetCurrent.vi"("Enabled?"=TRUE, "error in"=w47, "VISA resource name"=refnum<visa-resource-name> "COM8", "Function select"=enum16{"Init", "Set", "Close"}."Init", "current /mA"=w41) -> ("error out"=w46:errorcluster)  [unwired: 4 in, 2 out]
      n55 = flat-sequence {
        tunnel: [errorcluster {"status"=FALSE, "code"=0, "source"=""} ("error out")] -> w63
        tunnel: w59 -> [_]
        frame #0 {
        }
      }
      n56 = global write "GlobalExp.vi" "GlobalExp"(w107) -> ()
      n57 = Set Menu Item Info(7:"PMT_LARGE_VIEW" ("item tag"), 9:FALSE ("enabled"), 11:w87) -> (3:w82:refnum<k9>)  [unwired: 4 in, 1 out]
      n58 = disable-structure shown="FPGA_ENABLED==TRUE" {
        disable-tunnel: w63 -> [w124 w153]
        disable-tunnel: [w123 w153] -> w62
        frame condition #0 (active) {
          n59 = disable-structure shown="EXPERIMENT==MACRO, Default" {
            disable-tunnel: w124 -> [w152]
            disable-tunnel: [w129] -> w123
            disable-tunnel: "FPGA address" -> [w125]
            frame condition #0 (active) {
              n60 = xnode "Open FPGA VI Reference"("error in"=w152, "resource name"=w125) -> ("FPGA VI Reference Out"=w144:refnum<k20>, "error out"=w142:errorcluster)
              n61 = Multiply(x=3277, y=0.22) -> (x*y=w138:dbl)
              n62 = To Word Integer(number=w138) -> (16bit integer=w137:i16)
              n63 = xnode "Read/Write Control"("FPGA VI Reference In"=w144, "error in"=w142, "AO4 max"=w137) -> ("FPGA VI Reference Out"=w143:refnum<k20>, "error out"=w141:errorcluster)
              n64 = xnode "Invoke Method"("FPGA VI Reference In"=w143, "error in"=w141, "Requested Depth"=u32 100000) -> ("FPGA VI Reference Out"=w149:refnum<k20>, "error out"=w150:errorcluster)  [unwired: 1 out]
              n65 = local read "RSNPRZsettings"() -> (w128:T12)
              n66 = call "FPGAref.vi"("error in"=w150, "Enum"=enum16{"Set", "Get"}."Set", "FPGA VI Reference Out"=w149) -> ("error out"=w147:errorcluster)  [unwired: 3 in, 1 out]
              n67 = local read "AOMsetting"() -> (w136:T23)
              n68 = local read "DIOcluster"() -> (w145:T14)
              n69 = Unbundle By Name(w128) -> ("Average Counts :"=w127:dbl)
              n70 = call "FPGAinit.vi"("error in"=w147, "XAOMsetting"=w136, "DIOcluster"=w145) -> ("error out"=w134:errorcluster)  [unwired: 8 in]
              n71 = Unbundle By Name(w134) -> ("status"=w146:bool)
              n72 = local write "FPGAerr"(w146) -> ()
              n73 = call "AOMReadWrite.vi"("Enum"=enum16{"READ", "WRITE"}."WRITE", "error in"=w134) -> ("error out"=w133:errorcluster)  [unwired: 7 in, 2 out]
              n74 = call "Volt2Level.vi"("voltage /V"=w127) -> ("level"=w126:i16)
              n75 = call "FPGAref.vi"("error in"=w133, "Enum"=enum16{"Set", "Get"}."Get") -> ("error out"=w130:errorcluster, "FPGA VI Reference Out 2"=w131:refnum<k20>)  [unwired: 4 in]
              n76 = xnode "Read/Write Control"("FPGA VI Reference In"=w131, "error in"=w130, "AO5"=w126) -> ("error out"=w129:errorcluster)  [unwired: 1 out]
            }
          }
        }
        frame condition #1 {
        }
      }
      n77 = flat-sequence {
        tunnel: [errorcluster {"status"=FALSE, "code"=0, "source"=""} ("error out")] -> w49
        tunnel: w46 -> [_]
        frame #0 {
        }
      }
      n78 = Set Menu Item Info(7:"STOP_PMT" ("item tag"), 9:FALSE ("enabled"), 11:w82) -> (3:w81:refnum<k9>)  [unwired: 4 in, 1 out]
      n79 = local read "Param Cfg Path"() -> (w116:path)
      n80 = shared-variable "My Computer\\Global.lvlib\\Stop"(FALSE ("Stop")) -> ()  [unwired: 1 in, 1 out]
      n81 = local read "Connection Status"() -> (w50:T17)
      n82 = Set Menu Item Info(7:"STOP_CAMERA" ("item tag"), 9:FALSE ("enabled"), 11:w81) -> ()  [unwired: 4 in, 2 out]
      n83 = call "ParameterCfgLoad.vi"("Section"="ion_1", "configuration file path"=w116) -> ("section names list"=w115:string[], "Array - String"=w117:string[][])
      n84 = call "ConnectAtlas.vi"("error in (no error)"=w49) -> ("Atlas connection"=w38:bool, "AtlatsStat"=w39:string[], "Laser status"=w40:bool[])  [unwired: 8 in]
      n85 = local write "ParamCfgList"(w117) -> ()
      n86 = property on="ConfigHeader" class="CmbBox"("Strings[]"=w115) -> ()  [unwired: 2 in, 2 out]
      n87 = local write "AtlatsStat"(w39) -> ()
      n88 = local write "Laser status"(w40) -> ()
      n89 = control-ref of="AOMsetting"() -> (w61:refnum<vi>)
      n90 = property class="XAOMsetting (strict)"(reference=w61, "DisabledEnum"=w60) -> ()  [unwired: 1 in, 2 out]
      n91 = Bundle By Name(cluster=w50, "Atlas"=w38) -> (w109:T17)
      n92 = local read "Compiler Settings"() -> (w71:T18)
      n93 = control-ref of="Small Camera"() -> (w91:refnum<vi>)
      n94 = property class="IntGraph (strict)"(reference=w91, "DisabledEnum"=w60) -> ()  [unwired: 1 in, 2 out]
      n95 = local read "File Paths"() -> (w113:T19)
      n96 = call "CompilerLoadPulseTexts.vi"("compile settings"=w71) -> ("AuxCode 2"=w69:string, "MetaCode 2"=w70:string, "Maincode 2"=w72:string)  [unwired: 2 in]
      n97 = Unbundle By Name(w113) -> ("Local Save Path"=w112:path, "LocalSave"=w111:bool, "Newton Save Path"=w110:path)
      n98 = local write "MetaPulseCode"(w70) -> ()
      n99 = local write "MainPulsecode"(w72) -> ()
      n100 = local write "AuxPulseCode"(w69) -> ()
      n101 = control-ref of="PMT chart"() -> (w92:refnum<vi>)
      n102 = property class="WFChart (strict)"(reference=w92, "DisabledEnum"=w60) -> ()  [unwired: 1 in, 2 out]
      n103 = global write "DataLock.vi" "Lock"(FALSE ("Lock")) -> ()
      n104 = stacked-sequence {
        tunnel: w112 -> [_ w179 _ _]
        tunnel: w111 -> [_ w178 _ _]
        tunnel: w110 -> [w176 w177 _ _]
        tunnel: w109 -> [w174 _ _ _]
        tunnel: [_ _ _ errorcluster {"status"=FALSE, "code"=0, "source"=""} ("error constant")] -> w54
        frame #0 {
          n105 = call <vilib>:"Check if File or Folder Exists.vi"("path"=w176) -> ("file or folder exists?"=w175:bool)  [unwired: 8 in, 2 out]
          n106 = Bundle By Name(cluster=w174, "Newton"=w175) -> ()  [unwired: 1 out]
        }
        frame #1 {
          n107 = Get Date/Time In Seconds() -> (seconds since 1Jan1904=w186:timestamp)
          n108 = Select(t=w179, s=w178, f=w177) -> (s? t:f=w185:path)
          n109 = Format Date/Time String(time format string (%c)="%y%m%d", seconds (now)=w186) -> (date/time string=w184:string)  [unwired: 1 in]
          n110 = Build Path(base path=w185, name or relative path=w184) -> (appended path=w183:path)
          n111 = call <vilib>:"Check if File or Folder Exists.vi"("path"=w183) -> ("error out"=w181:errorcluster, "file or folder exists?"=w182:bool, "dup path"=w180:path)  [unwired: 8 in]
          n112 = case shown="False" w182 {
            tunnel: w181 -> [w190 _]
            tunnel: w180 -> [w189 _]
            frame False {
              n113 = Create Folder(path (use dialog)=w189, error in=w190) -> (error out=w188:errorcluster)  [unwired: 1 in, 2 out]
              n114 = case shown="Error" w188 {
                frame No Error {
                }
                frame Error {
                  n115 = call "LogWriteToGlobal.vi"("in string"="Error loading/creating data folder: invalid path.") -> ()  [unwired: 11 in]
                }
              }
            }
            frame True {
            }
          }
        }
        frame #2 {
          n116 = global write "GlobalExp.vi" "GlobalExp"(T31 {"Main Steps"=0.0, "Main Runs"=0.0, "ExpStatus"=enum."Idle", "Main Current Step"=0.0, "ExpNum"=0.0, "NewData"=FALSE, "date"="", "command"="", "Stop"=FALSE, "Pause"=FALSE, "Mathematica"="", "Main/Meta"=FALSE, "UpdateMath"=FALSE, "Camera"=FALSE, "MetaExpOver"=FALSE, "NextMetaExp"=FALSE} ("GlobalExp")) -> ()
        }
        frame #3 {
          n117 = local read "File Paths"() -> (w194:T19)
          n118 = call "InfoFile2ExpNum.vi"("File Paths"=w194) -> ("ExpNum string"=w195:string)  [unwired: 10 in]
          n119 = local write "ExpNumIndicator"(w195) -> ()
          n120 = disable-structure shown="Disabled" {
            frame Disabled {
              n121 = call "ExpLogInit.vi"() -> ()  [unwired: 12 in]
            }
            frame Enabled {
            }
          }
        }
      }
      n122 = flat-sequence {
        tunnel: [errorcluster {"status"=FALSE, "code"=0, "source"=""} ("error out")] -> w96
        tunnel: w62 -> [_]
        frame #0 {
        }
      }
      n123 = local read "Tab control"() -> (w95:cluster{"visible":bool, "Tab name":string}[])
      n124 = local read "Large cam coords"() -> (w80:T11)
      n125 = control-ref of="MasterTabCtl"() -> (w97:refnum<vi>)
      n126 = disable-structure shown="Disabled" {
        frame Disabled {
          n127 = Current VI's Path() -> (path=w203:path)
          n128 = Open VI Reference(vi path=w203) -> (vi reference=w202:refnum<vi>, error out=w201:errorcluster)  [unwired: 5 in]
          n129 = property class="VI"(reference=w202, error in=w201, "Front Panel.WinBounds"=T32 {"Left"=2, "Top"=70, "Right"=1901, "Bottom"=1021} ("Front Panel Window:Panel Bounds")) -> (reference out=w199:refnum<vi>, error out=w198:errorcluster)
          n130 = property class="VI"(reference=w199, error in=w198) -> (error out=w196:errorcluster, "Panel"=w197:refnum<vi>)  [unwired: 1 out]
          n131 = property class="Pnl" props=["Panes[]"](reference=w197, error in=w196) -> ()  [unwired: 3 out]
        }
        frame Enabled {
        }
      }
      n132 = call "TabVisibilityControl.vi"("error in (no error)"=w96, "Tab Control 2"=w97, "Tab control"=w95) -> ("error out"=w57:errorcluster, "Running VIs ref"=→"Running VIs ref":refnum<vi>[])  [unwired: 7 in]
      n133 = Unbundle By Name(w80) -> ("Top :"=w76:dbl, "Bottom :"=w75:dbl, "Left :"=w74:dbl, "Right :"=w73:dbl)
      n134 = flat-sequence {
        tunnel: [errorcluster {"status"=FALSE, "code"=0, "source"=""} ("error out")] -> _
        tunnel: w57 -> [_]
        frame #0 {
        }
      }
      n135 = Bundle By Name(cluster=w77, "min"=w75, "max"=w76) -> (w79:cluster{"min":i16, "max":i16})
      n136 = Bundle By Name(cluster=w77, "min"=w74, "max"=w73) -> (w78:cluster{"min":i16, "max":i16})
      n137 = local read "TreeFolderPath"() -> (w65:path)
      n138 = property on="CamYSlider" class="XVerticalSlide (strict)"("Property"=w79) -> ()  [unwired: 2 in, 2 out]
      n139 = property on="CamXSlide" class="XHorizontalSlide (strict)"("Property"=w78) -> ()  [unwired: 2 in, 2 out]
      n140 = control-ref of="DataTree"() -> (w64:refnum<vi>)
      n141 = local write "DisconnectCamera"(FALSE ("DisconnectCamera")) -> ()
      n142 = call "ExplorerTreeUpdate.vi"("Tree ref"=w64, "Folder Path"=w65) -> ()  [unwired: 10 in]
      n143 = local read "ArbitraryWaveListMW"() -> (w53:dbl[][])
      n144 = call "AWGCompileContinuousWave.vi"("error in"=w54, "ArbitraryWaveListMW"=w53) -> ("error out"=w56:errorcluster, "array MW and RF"=w55:variant[])
      n145 = call "AWGSendPulseArrayContinuous.vi"("error in (no error)"=w56, "AWG pulses array"=w55) -> ("error out"=w52:errorcluster)  [unwired: 8 in, 1 out]
    }
    frame #2 {
      # "Main program loops"
      n146 = while {
        stop <- w549 stop-if-true
        # "Global Logic and Updates"
        n147 = disable-structure shown="Enabled" {
          frame Enabled {
            n148 = local read "Connection Status"() -> (w553:T17)
            n149 = Unbundle By Name(w553) -> ("Atlas"=w552:bool)
            n150 = case shown="True" w552 {
              frame False {
              }
              frame True {
                n151 = call "AtlasWavelengths.vi"() -> ("error out"=w554:errorcluster, "AtlasStat"=w555:string[], "Wavelengths"=w557:dbl[], "Laser status"=w558:bool[])  [unwired: 8 in]
                n152 = case shown="No Error" w554 {
                  tunnel: w558 -> [w572 _]
                  tunnel: w557 -> [w571 _]
                  tunnel: "369 unlock notification" -> [w560 _]
                  tunnel: w555 -> [w559 _]
                  frame No Error {
                    n153 = local write "Laser status"(w572) -> ()
                    n154 = local write "AtlatsStat"(w559) -> ()
                    n155 = Array To Cluster(array=w571) -> (cluster=w570:T35)
                    n156 = Unbundle(w570) -> ("Wavelengths[0]"=w563:dbl, "Wavelengths[1]"=w562:dbl, "Wavelengths[2]"=w561:dbl)  [unwired: 6 out]
                    n157 = local read "399 cluster"() -> (w566:T1)
                    n158 = in-place {
                      in-place-border: w563 -> [w575]
                      n159 = in-place-cluster #2(w566) -> ()  [unwired: 1 out]
                      n160 = in-place-cluster #2("wavelength"=w575) -> (w567:T1)
                    }
                    n161 = local read "935 cluster"() -> (w565:T1)
                    n162 = in-place {
                      in-place-border: w562 -> [w574]
                      n163 = in-place-cluster #3(w565) -> ()  [unwired: 1 out]
                      n164 = in-place-cluster #3("wavelength"=w574) -> (w564:T1)
                    }
                    n165 = local read "739 cluster"() -> (w569:T1)
                    n166 = in-place {
                      in-place-border: w561 -> [w576]
                      n167 = in-place-cluster #4(w569) -> ()  [unwired: 1 out]
                      n168 = in-place-cluster #4("wavelength"=w576) -> (w568:T1)
                    }
                    n169 = case shown="True" w560 {
                      tunnel: w561 -> [_ w573]
                      frame False {
                      }
                      frame True {
                        n170 = call "LaserUnlockNotification.vi"("369wavelength"=w573) -> ()  [unwired: 11 in]
                      }
                    }
                    n171 = local write "935 cluster"(w564) -> ()
                    n172 = local write "739 cluster"(w568) -> ()
                    n173 = local write "399 cluster"(w567) -> ()
                  }
                  frame Error {
                  }
                }
              }
            }
          }
          frame Disabled {
          }
        }
        n174 = local read "Pause/Stop"() -> (w539:cluster{"Exp Stop":bool, "Pause":bool})
        n175 = Unbundle By Name(w539) -> ("Exp Stop"=w538:bool, "Pause"=w540:bool)
        n176 = global read "GlobalPyConsole.vi" "Python Console"() -> (w534:string)
        n177 = global read "GlobalExp.vi" "GlobalExp"() -> (w541:T31)
        n178 = local write "Python Console"(w534) -> ()
        n179 = Unbundle By Name(w541) -> ("ExpStatus"=w543:T29, "Stop"=w537:bool)
        n180 = Or(x=w537, y=w538) -> (x .or. y?=w536:bool)
        n181 = Bundle By Name(cluster=w541, "Pause"=w540, "Stop"=w536) -> (w535:T31)
        n182 = global write "GlobalExp.vi" "GlobalExp"(w535) -> ()
        n183 = local read "Stop button"() -> (w551:bool)
        n184 = shared-variable ".\\Global.lvlib\\GlobalLog"() -> (w545:string)  [unwired: 1 in, 1 out]
        n185 = local write "GlobalLog"(w545) -> ()
        n186 = Equal?(x=T29."Idle", y=w543) -> (x = y?=w546:bool)
        n187 = case shown="\"Idle\", Default" w543 {
          tunnel: [cluster{u32, u32}[] [{51225, 51225}] cluster{u32, u32}[] [{16860, 16860}] cluster{u32, u32}[] [{16860, 16860}] cluster{u32, u32}[] [{13971251, 13971251}] cluster{u32, u32}[] [{16751616, 16751616}]] -> w547
          frame "Idle", Default {
          }
          frame "MainRunning" {
          }
          frame "AuxRunning" {
          }
          frame "Stop" {
          }
          frame "Innit" {
          }
        }
        n188 = Compound Arithmetic op=OR(w551) -> (w550:bool)
        n189 = And(x=w546, y=w550) -> (x .and. y?=w549:bool)
        n190 = shared-variable ".\\Global.lvlib\\ExperimentLog"() -> (w544:string)  [unwired: 1 in, 1 out]
        n191 = case shown="True" w549 {
          selector: w549 -> [_ w582]
          tunnel: w549 -> [_ _]
          frame False {
          }
          frame True {
            n192 = shared-variable "My Computer\\Global.lvlib\\Stop"(w582) -> ()  [unwired: 1 in, 1 out]
          }
        }
        n193 = local write "ExpLog"(w544) -> ()
        n194 = property on="Stop button" class="Bool (strict)"("Colors [4]"=w547) -> ()  [unwired: 2 in, 2 out]
        n195 = Wait (ms)(milliseconds to wait=u32 100) -> ()  [unwired: 1 out]
      }
      n196 = while {
        stop <- w208 stop-if-true
        # "Camera"
        n197 = global read "GlobalImagingStatus.vi" "ImagingStatus"() -> (w206:T27)
        n198 = Equal?(x=w206, y=ImagingStatusControl."Camera") -> (x = y?=w207:bool)
        n199 = case shown="True" w207 {
          frame False {
            n200 = Wait (ms)(milliseconds to wait=u32 50) -> ()  [unwired: 1 out]
          }
          frame True {
            n201 = call "CameraCheckUpdate.vi"() -> ("error constant 2"=w220:errorcluster)  [unwired: 11 in]
            n202 = disable-structure shown="CAMERA_SIMULATED==FALSE" {
              disable-tunnel: w220 -> [w224 w227]
              disable-tunnel: [w223 w228] -> w218
              disable-tunnel: enum16{"Start", "Stop", "Acquire", "Update"}."Acquire" ("Enum") -> [w222 w226]
              disable-tunnel: [w221 w225] -> w216
              frame condition #0 {
                n203 = call "CameraCtrlDEBUG.vi"("error constant"=w224, "Enum"=w222) -> ("error constant 2"=w221:errorcluster, "Large Camera"=w223:dbl[][])  [unwired: 8 in]
              }
              frame condition #1 (active) {
                n204 = call "CameraCtrl.vi"("error constant"=w227, "Enum"=w226) -> ("error constant 2"=w225:errorcluster, "Large Camera"=w228:i32[][])  [unwired: 7 in, 1 out]
              }
            }
            n205 = local read "Large cam coords"() -> (w215:T11)
            n206 = control-ref of="Left ion graph"() -> (w211:refnum<vi>)
            n207 = control-ref of="Big Camera"() -> (w217:refnum<vi>)
            n208 = control-ref of="Small Camera"() -> (w212:refnum<vi>)
            n209 = control-ref of="CamXSlide"() -> (w214:refnum<vi>)
            n210 = control-ref of="CamYSlider"() -> (w213:refnum<vi>)
            n211 = local read "ion coords"() -> (w210:T11)
            n212 = call "CameraReshapeViews.vi"("Cam img in"=w218, "XHorizontalSlide"=w214, "XVerticalSlide"=w213, "Large Cam ref"=w217, "Small cam ref"=w212, "Ions cam ref"=w211, "error in (no error)"=w216, "Large cam coords"=w215, "ion coords"=w210) -> ()  [unwired: 6 in, 1 out]
          }
        }
        n213 = shared-variable "My Computer\\Global.lvlib\\Stop"() -> (w208:bool)  [unwired: 1 in, 1 out]
      }
      n214 = while {
        shift-right: [w232] -> _
        shift-left: FALSE -> [w231]
        stop <- w229 stop-if-true
        # "Meta/Queue Py Client"
        n215 = control-ref of="QueueControl"() -> (w230:refnum<vi>)
        n216 = shared-variable "My Computer\\Global.lvlib\\Stop"() -> (w229:bool)  [unwired: 1 in, 1 out]
        n217 = global read "GlobalExp.vi" "GlobalExp"() -> (w234:T31)
        n218 = Unbundle By Name(w234) -> ("Main/Meta"=w233:bool)
        n219 = case shown="True" w233 {
          selector: w233 -> [w235 w244]
          tunnel: [w235 w244] -> w232
          tunnel: w231 -> [w237 _]
          tunnel: w230 -> [w236 w243]
          frame False {
            n220 = case shown="True" w237 {
              tunnel: w236 -> [_ w242]
              frame False {
              }
              frame True {
                n221 = call "MetaClientQueueTCP.vi"("Enum"=enum16{"shutdown", "send_queue", "get_queue"}."shutdown", "RefIn"=w242) -> ("error out"=w239:errorcluster)  [unwired: 8 in, 1 out]
                n222 = call "MetaClientCont.vi"("error in (no error)"=w239, "Action"=enum16{"Run", "Exit"}."Exit") -> ("error out"=w238:errorcluster)  [unwired: 8 in, 1 out]
                n223 = call "KillAllOpenCMD.vi"("error in (no error)"=w238) -> ()  [unwired: 10 in, 1 out]
              }
            }
          }
          frame True {
            n224 = local read "QueueControl"() -> (w246:T3)
            n225 = event shown="[0] Timeout" {
              selector: _ -> [_ _ _ _ _ _ _ _ _]
              dyn-events: _ -> [_ _ _ _ _ _ _ _ _]
              timeout: 500 -> [_ _ _ _ _ _ _ _ _]
              tunnel: w243 -> [w248 _ w258 _ w266 w271 w276 w281 w290]
              tunnel: w246 -> [_ _ _ w263 _ _ _ _ _]
              event Timeout {
                n226 = event-data() -> ()  [unwired: 1 in, 3 out]
                n227 = local read "QueueChanged"() -> (w250:bool)
                n228 = case shown="False" w250 {
                  tunnel: [enum16{"shutdown", "send_queue", "get_queue"}."get_queue" ("Enum") enum16{"shutdown", "send_queue", "get_queue"}."send_queue" ("Enum")] -> w251
                  frame False {
                  }
                  frame True {
                    n229 = local write "QueueChanged"(FALSE ("QueueChanged")) -> ()
                  }
                }
                n230 = call "MetaClientQueueTCP.vi"("Enum"=w251, "RefIn"=w248) -> ("RefOut"=w247:refnum<vi>)  [unwired: 8 in, 1 out]
                n231 = call "QueueControl.vi"("Enum"=T33."update", "RefIn"=w247) -> ()  [unwired: 10 in]
              }
              event Value Change {
                n232 = event-data() -> ("NewVal"=w257:string)  [unwired: 1 in]
                n233 = local read "QueueControl"() -> (w256:T3)
                n234 = Bundle By Name(cluster=w256, "Add To Queue:"=w257) -> (w255:T3)
                n235 = local write "QueueControl"(w255) -> ()
              }
              event Value Change {
                n236 = event-data() -> ("NewVal"=w259:bool)  [unwired: 1 in]
                n237 = case shown="True" w259 {
                  tunnel: w258 -> [_ w261]
                  frame False {
                  }
                  frame True {
                    n238 = local write "QueueChanged"(TRUE ("QueueChanged")) -> ()
                    n239 = call "QueueControl.vi"("Enum"=T33."top", "RefIn"=w261) -> ()  [unwired: 10 in]
                  }
                }
              }
              event Value Change {
                n240 = event-data() -> ("NewVal"=w265:i32)  [unwired: 1 in]
                n241 = Bundle By Name(cluster=w263, "QueueFromServer"=w265) -> (w264:T3)
                n242 = local write "QueueControl"(w264) -> ()
              }
              event Value Change {
                n243 = event-data() -> ("NewVal"=w267:bool)  [unwired: 1 in]
                n244 = case shown="True" w267 {
                  tunnel: w266 -> [_ w268]
                  frame False {
                  }
                  frame True {
                    n245 = local write "QueueChanged"(TRUE ("QueueChanged")) -> ()
                    n246 = call "QueueControl.vi"("Enum"=T33."up", "RefIn"=w268) -> ()  [unwired: 10 in]
                  }
                }
              }
              event Value Change {
                n247 = event-data() -> ("NewVal"=w272:bool)  [unwired: 1 in]
                n248 = case shown="True" w272 {
                  tunnel: w271 -> [_ w274]
                  frame False {
                  }
                  frame True {
                    n249 = local write "QueueChanged"(TRUE ("QueueChanged")) -> ()
                    n250 = call "QueueControl.vi"("Enum"=T33."down", "RefIn"=w274) -> ()  [unwired: 10 in]
                  }
                }
              }
              event Value Change {
                n251 = event-data() -> ("NewVal"=w277:bool)  [unwired: 1 in]
                n252 = case shown="True" w277 {
                  tunnel: w276 -> [_ w279]
                  frame False {
                  }
                  frame True {
                    n253 = local write "QueueChanged"(TRUE ("QueueChanged")) -> ()
                    n254 = call "QueueControl.vi"("Enum"=T33."bot", "RefIn"=w279) -> ()  [unwired: 10 in]
                  }
                }
              }
              event Value Change {
                n255 = event-data() -> ("NewVal"=w282:bool)  [unwired: 1 in]
                n256 = case shown="True" w282 {
                  tunnel: w281 -> [_ w284]
                  frame False {
                  }
                  frame True {
                    n257 = local write "QueueChanged"(TRUE ("QueueChanged")) -> ()
                    n258 = call "QueueControl.vi"("Enum"=T33."del", "RefIn"=w284) -> ()  [unwired: 10 in]
                  }
                }
              }
              event Value Change {
                n259 = event-data() -> ("NewVal"=w291:string)  [unwired: 1 in]
                n260 = property class="Clust (strict)"(reference=w290) -> (reference out=w288:refnum<vi>, "Value"=w289:T3)  [unwired: 1 in, 1 out]
                n261 = case shown="\"freqscan\", Default" w291 {
                  tunnel: ["freqscan(\"plus1\", -4, 1, 9, 200)" "timescan(\"dressingP1ms\", 100, 8, 8, 200)"] -> w286
                  frame "freqscan", Default {
                  }
                  frame "timescan" {
                  }
                }
                n262 = in-place {
                  in-place-border: w286 -> [w292]
                  n263 = in-place-cluster #5(w289) -> ()  [unwired: 1 out]
                  n264 = in-place-cluster #5("Add To Queue:"=w292) -> (w287:T3)
                }
                n265 = property class="Clust (strict)"(reference=w288, "Value"=w287) -> ()  [unwired: 1 in, 2 out]
              }
            }
          }
        }
      }
      n266 = while {
        stop <- _ stop-if-true
      }
      n267 = while {
        stop <- w583 stop-if-true
        # "Pulse Programming Tab, Runtime Menu"
        n268 = shared-variable "My Computer\\Global.lvlib\\Stop"() -> (w583:bool)  [unwired: 1 in, 1 out]
        n269 = local read "Param Cfg Path"() -> (w584:path)
        n270 = local read "ParamCfgList"() -> (w586:string[][])
        n271 = local read "ConfigHeader"() -> (w585:string)
        n272 = event shown="[0] Timeout" {
          selector: _ -> [_ _ _ _ _ _ _ _ _ _ _ _ _ _ _ _ _ _ _ _ _ _ _ _ _ _ _ _ _ _]
          dyn-events: _ -> [_ _ _ _ _ _ _ _ _ _ _ _ _ _ _ _ _ _ _ _ _ _ _ _ _ _ _ _ _ _]
          timeout: 50 -> [_ _ _ _ _ _ _ _ _ _ _ _ _ _ _ _ _ _ _ _ _ _ _ _ _ _ _ _ _ _]
          tunnel: w586 -> [_ _ _ _ _ w628 w635 _ _ _ _ _ _ _ _ _ _ _ _ _ _ _ _ _ _ _ _ _ _ _]
          tunnel: w585 -> [_ _ _ _ _ _ w636 _ w644 _ _ _ _ _ _ _ _ _ _ _ _ _ _ _ _ _ _ _ _ _]
          tunnel: w584 -> [_ _ _ _ _ w624 w637 _ w643 _ _ _ _ _ _ _ _ _ _ _ _ _ _ _ _ _ _ _ _ _]
          event Timeout {
            w588 = FALSE ("MainLoad")
            n273 = event-data() -> ()  [unwired: 1 in, 3 out]
            n274 = global read "GlobalExp.vi" "GlobalExp"() -> (w594:T31)
            n275 = local write "AuxSave"(w588) -> ()
            n276 = local write "MainSave"(w588) -> ()
            n277 = local write "MainLoad"(w588) -> ()
            n278 = local write "MainCompile"(w588) -> ()
            n279 = local write "LoadExpLog"(w588) -> ()
            n280 = local write "SaveExpLog"(w588) -> ()
            n281 = Unbundle By Name(w594) -> ("ExpNum"=w589:dbl)
            n282 = Format Into String(format string="%03d", w589) -> (resulting string=w596:string)  [unwired: 2 in, 1 out]
            n283 = local write "MetaPush"(w588) -> ()
            n284 = local write "Process Statedet"(w588) -> ()
            n285 = local write "AuxLoad"(w588) -> ()
            n286 = local write "AuxCompile"(w588) -> ()
            n287 = local write "MetaLoad"(w588) -> ()
            n288 = local write "MetaSave"(w588) -> ()
            n289 = Concatenate Strings("Experiment #: " ("string"), w596) -> (w597:string)
            n290 = local write "ExpNumIndicator"(w597) -> ()
            n291 = local write "DisplayImage"(w588) -> ()
            n292 = local write "Find Probabilites"(w588) -> ()
            n293 = local write "Analyze Probs"(w588) -> ()
            n294 = local read "MathImageCtl"() -> (w591:T5)
            n295 = disable-structure shown="Disabled" {
              frame Disabled {
                n296 = local read "VISA: Pressure"() -> (w600:refnum<visa-resource-name>)
                n297 = call "DriverVarianXGS-600.vi"("VISA resource name"=w600, "Action"=enum16{"Start", "Read", "Stop"}."Read") -> ("Pressure"=w599:dbl)  [unwired: 1 in, 3 out]
                n298 = local write "Pressure"(w599) -> ()
              }
              frame Enabled {
              }
            }
            n299 = Bundle By Name(cluster=w591, "Reload"=FALSE ("Auto :")) -> (w592:T5)
            n300 = local write "MathImageCtl"(w592) -> ()
            n301 = local write "LoadPulseSeq"(w588) -> ()
          }
          event "Run TDC": Value Change {
            n302 = event-data() -> ()  [unwired: 1 in, 6 out]
            n303 = local read "N measurements"() -> (w603:dbl)
            n304 = local write "Run TDC"(FALSE ("Run TDC")) -> ()
            n305 = call "FPGAref.vi"("Enum"=enum16{"Set", "Get"}."Get") -> ("FPGA VI Reference Out 2"=w604:refnum<k20>)  [unwired: 5 in, 1 out]
            n306 = call-poly <vilib>:"Write Delimited Spreadsheet.vi"("1D data"=i32[] [0]) -> ("new file path (Not A Path if cancelled)"=w601:path)  [unwired: 13 in, 1 out]
            n307 = for {
              N: w603 -> [_]
              tunnel: w604 -> [w618]
              shift-right: [w608] -> _
              shift-left: w601 -> [w609]
              i -> [w612]
              stop <- "Stop" stop-if-true
              n308 = local write "Current iteration"(w612) -> ()
              n309 = xnode "Read/Write Control"("FPGA VI Reference In"=w618, "Acquire times"=TRUE, "N photons"=u32 50) -> ("FPGA VI Reference Out"=w617:refnum<k20>)  [unwired: 1 in, 1 out]
              n310 = To Unsigned Long Integer(number=50) -> (unsigned 32bit integer=w615:u32)
              n311 = xnode "Invoke Method"("FPGA VI Reference In"=w617, "Number of Elements"=w615, "Timeout (ms)"=10000) -> ("Data"=w613:u32[])  [unwired: 1 in, 3 out]
              n312 = for {
                tunnel: w613 -> [w622] mode=indexing
                tunnel: [w622] -> w610 mode=indexing if=w621
                n313 = Not Equal To 0?(x=w622) -> (x != 0?=w621:bool)
              }
              n314 = local write "Waveform Chart"(w610) -> ()
              n315 = call-poly <vilib>:"Write Delimited Spreadsheet.vi"("file path (dialog if empty)"=w609, "1D data"=w610, "append to file? (new file:F)"=TRUE) -> ("new file path (Not A Path if cancelled)"=w608:path)  [unwired: 11 in, 1 out]
            }
          }
          event "LoadExpLog": Value Change {
            n316 = event-data() -> ()  [unwired: 1 in, 6 out]
            n317 = call "ExpLogLoad.vi"() -> ()  [unwired: 12 in]
          }
          event "SaveExpLog": Value Change {
            n318 = event-data() -> ()  [unwired: 1 in, 6 out]
            n319 = call "ExpLogSave.vi"() -> ()  [unwired: 12 in]
          }
          event "MetaPush": Value Change {
            n320 = event-data() -> ()  [unwired: 1 in, 6 out]
            n321 = local read "MetaPulseCode"() -> (w623:string)
            n322 = call "MetaPushScript.vi"("MetaScript"=w623) -> ()  [unwired: 11 in]
          }
          event "ConfigHeader": Value Change {
            n323 = event-data() -> ("OldVal"=w625:string, "NewVal"=w626:string)  [unwired: 1 in]
            n324 = stacked-sequence {
              tunnel: w625 -> [w631 _]
              tunnel: w628 -> [w630 _]
              tunnel: w626 -> [_ w634]
              tunnel: w624 -> [w629 w633]
              tunnel: [_ w632] -> w627
              frame #0 {
                n325 = call "ParameterCfgSave.vi"("config_values"=w630, "section"=w631, "appended path"=w629) -> ()
              }
              frame #1 {
                n326 = call "ParameterCfgLoad.vi"("Section"=w634, "configuration file path"=w633) -> ("Array - String"=w632:string[][])  [unwired: 1 out]
              }
            }
            n327 = local write "ParamCfgList"(w627) -> ()
          }
          event "Param Cfg Save": Value Change {
            n328 = event-data() -> ()  [unwired: 1 in, 1 out]
            n329 = call "ParameterCfgSave.vi"("config_values"=w635, "section"=w636, "appended path"=w637) -> ()
          }
          event "UpdateAWGSeqGraph": Value Change {
            n330 = event-data() -> ("NewVal"=w638:bool)  [unwired: 1 in, 5 out]
            n331 = case shown="True" w638 {
              frame False {
              }
              frame True {
                n332 = control-ref of="AWGgraph"() -> (w639:refnum<vi>)
                n333 = local read "MW sequence array"() -> (w641:T9[])
                n334 = local read "RF sequence array"() -> (w640:T9[])
                n335 = call "UpdateAWGGraph.vi"("RF Sequence array"=w640, "MW sequence array"=w641, "Waveform Graph 2"=w639) -> ()  [unwired: 9 in]
              }
            }
          }
          event "Param Cfg Load": Value Change {
            n336 = event-data() -> ()  [unwired: 1 in, 1 out]
            n337 = call "ParameterCfgLoad.vi"("Section"=w644, "configuration file path"=w643) -> ("Array - String"=w642:string[][])  [unwired: 1 out]
            n338 = local write "ParamCfgList"(w642) -> ()
          }
          event "MainCompile": Value Change {
            n339 = event-data() -> ("NewVal"=w645:bool)  [unwired: 1 in]
            n340 = case shown="True" w645 {
              frame False {
              }
              frame True {
                n341 = flat-sequence {
                  frame #0 {
                    n342 = local read "MainPulsecode"() -> (w647:string)
                    n343 = call "SaveScriptFile.vi"("file name"="scriptmain.py", "text"=w647) -> ()  [unwired: 9 in, 1 out]
                  }
                  frame #1 {
                    n344 = local read "Compiler Settings"() -> (w654:T18)
                    n345 = call "CompileMaster.vi"("Type"=enum16{"Meta", "Aux", "Main"}."Main" ("Enum"), "Stepnum"=0, "Compiler Settings"=w654) -> ("CompileSuccess?"=w649:bool, "PulseList"=w652:T36[], "RF Array"=w648:variant[], "Standard Error Out"=w653:string)  [unwired: 1 in, 2 out]
                    n346 = local write "Python Console"(w653) -> ()
                    n347 = case shown="True" w649 {
                      tunnel: w652 -> [_ w659]
                      tunnel: w648 -> [_ w657]
                      frame False {
                      }
                      frame True {
                        n348 = call "CompileParseMWPulse.vi"("Pulse List In"=w659) -> ("Pulse seq out"=w658:T37)
                        n349 = call "CompileParseAWGPulse.vi"("RF Array"=w657) -> ("MWout"=w656:T9[], "RFout"=w655:T9[])
                        n350 = local write "MW sequence array"(w656) -> ()
                        n351 = local write "MainPulseSeq"(w658) -> ()
                        n352 = local write "RF sequence array"(w655) -> ()
                      }
                    }
                  }
                }
              }
            }
          }
          event Value Change {
            n353 = event-data() -> ()  [unwired: 1 in, 1 out]
            n354 = local read "File Paths"() -> (w661:T19)
            n355 = local read "MathImageCtl"() -> (w662:T5)
            n356 = control-ref of="PltPic"() -> (w660:refnum<vi>)
            n357 = call "UpdateMathsPic.vi"("ref pic in"=w660, "File Paths"=w661, "MathImageCtl"=w662) -> ("pic out"=w663:picture)  [unwired: 8 in]
            n358 = local write "PltPic"(w663) -> ()
          }
          event "SaveSession": Value Change {
            n359 = event-data() -> ()  [unwired: 1 in, 1 out]
            n360 = control-ref of="This VI"() -> (w664:refnum<vi>)
            n361 = local write "SaveSession"(FALSE ("SaveSession")) -> ()
            n362 = call "SessionCfgSave.vi"("This VI"=w664) -> ()  [unwired: 10 in, 1 out]
          }
          event "LoadSession": Value Change {
            n363 = event-data() -> ()  [unwired: 1 in, 6 out]
            n364 = control-ref of="This VI"() -> (w666:refnum<vi>)
            n365 = local write "LoadSession"(FALSE ("LoadSession")) -> ()
            n366 = call "SessionCfgLoad.vi"("This VI"=w666) -> ()  [unwired: 10 in, 1 out]
          }
          event "AuxCompile": Value Change {
            n367 = event-data() -> ("NewVal"=w668:bool)  [unwired: 1 in]
            n368 = case shown="True" w668 {
              frame False {
              }
              frame True {
                n369 = local read "Compiler Settings"() -> (w673:T18)
                n370 = call "CompileMaster.vi"("Type"=enum16{"Meta", "Aux", "Main"}."Aux", "Stepnum"=0, "Compiler Settings"=w673) -> ("PulseList"=w670:T36[], "Standard Error Out"=w671:string)  [unwired: 1 in, 4 out]
                n371 = local write "Python Console"(w671) -> ()
                n372 = call "CompileParseMWPulse.vi"("Pulse List In"=w670) -> ("Pulse seq out"=w669:T37)
                n373 = local write "AuxPulseSeq"(w669) -> ()
              }
            }
          }
          event "MainLoad": Value Change {
            n374 = event-data() -> ()  [unwired: 1 in, 2 out]
            n375 = call <vilib>:"Application Directory.vi"() -> ("Application Directory"=w678:path)
            n376 = Build Path(base path=w678, name or relative path="python") -> (appended path=w676:path)
            n377 = call "File Dialog"("start path"=w676, "pattern (all files)"="*.py") -> ("selected path"=w682:path, "error out"=w681:errorcluster)  [unwired: 10 in, 2 out]
            n378 = Unbundle By Name(w681) -> ("status"=w680:bool, "source"=w679:string)
            n379 = case shown="False" w680 {
              tunnel: w682 -> [w686 _]
              tunnel: [w685 ""] -> w675
              tunnel: w681 -> [w684 _]
              tunnel: w679 -> [_ w688]
              frame False {
                n380 = Read from Text File(file (use dialog)=w686, error in=w684) -> (text=w685:string)  [unwired: 2 in, 3 out]
              }
              frame True {
                n381 = local write "Python Console"(w688) -> ()
              }
            }
            n382 = local write "MainPulsecode"(w675) -> ()
          }
          event "AuxLoad": Value Change {
            n383 = event-data() -> ()  [unwired: 1 in, 2 out]
            n384 = call <vilib>:"Application Directory.vi"() -> ("Application Directory"=w691:path)
            n385 = Build Path(base path=w691, name or relative path="python") -> (appended path=w692:path)
            n386 = call "File Dialog2"("start path"=w692, "pattern (all files)"="*.py") -> ("selected path"=w696:path, "error out"=w695:errorcluster)  [unwired: 10 in, 2 out]
            n387 = Unbundle By Name(w695) -> ("status"=w694:bool, "source"=w693:string)
            n388 = case shown="False" w694 {
              tunnel: w696 -> [w700 _]
              tunnel: [w699 ""] -> w689
              tunnel: w695 -> [w698 _]
              tunnel: w693 -> [_ w702]
              frame False {
                n389 = Read from Text File(file (use dialog)=w700, error in=w698) -> (text=w699:string)  [unwired: 2 in, 3 out]
              }
              frame True {
                n390 = local write "Python Console"(w702) -> ()
              }
            }
            n391 = local write "AuxPulseCode"(w689) -> ()
          }
          event "MetaLoad": Value Change {
            n392 = event-data() -> ()  [unwired: 1 in, 1 out]
            n393 = call <vilib>:"Application Directory.vi"() -> ("Application Directory"=w706:path)
            n394 = Build Path(base path=w706, name or relative path="python\\pulse\\_metascripts") -> (appended path=w704:path)
            n395 = call "File Dialog6"("start path"=w704, "pattern (all files)"="*.*") -> ("selected path"=w710:path, "error out"=w709:errorcluster)  [unwired: 10 in, 2 out]
            n396 = Unbundle By Name(w709) -> ("status"=w708:bool, "source"=w707:string)
            n397 = case shown="False" w708 {
              tunnel: w710 -> [w714 _]
              tunnel: [w713 ""] -> w703
              tunnel: w709 -> [w712 _]
              tunnel: w707 -> [_ w716]
              frame False {
                n398 = Read from Text File(file (use dialog)=w714, error in=w712) -> (text=w713:string)  [unwired: 2 in, 3 out]
              }
              frame True {
                n399 = local write "Python Console"(w716) -> ()
              }
            }
            n400 = local write "MetaPulseCode"(w703) -> ()
          }
          event "MainSave": Value Change {
            n401 = event-data() -> ()  [unwired: 1 in, 6 out]
            n402 = local read "MainPulsecode"() -> (w719:string)
            n403 = call "SaveScriptFile.vi"("file name"="scriptmain.py", "text"=w719) -> ("source"=w718:string)  [unwired: 9 in]
            n404 = local write "Python Console"(w718) -> ()
          }
          event "AuxSave": Value Change {
            n405 = event-data() -> ()  [unwired: 1 in, 6 out]
            n406 = local read "AuxPulseCode"() -> (w722:string)
            n407 = call "SaveScriptFile.vi"("file name"="scriptaux.py", "text"=w722) -> ("source"=w721:string)  [unwired: 9 in]
            n408 = local write "Python Console"(w721) -> ()
          }
          event "MetaSave": Value Change {
            n409 = event-data() -> ()  [unwired: 1 in, 6 out]
            n410 = call <vilib>:"Application Directory.vi"() -> ("Application Directory"=w724:path)
            n411 = Build Path(base path=w724, name or relative path="python") -> (appended path=w726:path)
            n412 = call "File Dialog5"("start path"=w726, "pattern (all files)"="*.py") -> ("selected path"=w730:path, "error out"=w728:errorcluster)  [unwired: 10 in, 2 out]
            n413 = local read "MetaPulseCode"() -> (w723:string)
            n414 = Unbundle By Name(w728) -> ("status"=w729:bool, "source"=w731:string)
            n415 = case shown="True" w729 {
              tunnel: w730 -> [w733 _]
              tunnel: w723 -> [w732 _]
              tunnel: w731 -> [_ w734]
              frame False {
                n416 = Write to Text File(file (use dialog)=w733, text=w732) -> ()  [unwired: 2 in, 3 out]
              }
              frame True {
                n417 = local write "Python Console"(w734) -> ()
              }
            }
          }
          event Menu Selection (User) {
            n418 = event-data() -> ("ItemTag"=w735:string)  [unwired: 1 in]
            n419 = case shown="\"RUN_CAMERA\"" w735 {
              frame "False", Default {
              }
              frame "CAMERA_SETTINGS" {
                n420 = vi-ref "CameraSettingsMenu.vi"() -> (w738:refnum<vi>)
                n421 = call <vilib>:"Application Directory.vi"() -> ("Application Directory"=w740:path)
                n422 = Build Path(base path=w740, name or relative path="VIs\\Camera\\CameraSettingsMenu.vi") -> (appended path=w737:path)
                n423 = Open VI Reference(type specifier VI Refnum (for type only)=w738, vi path=w737, options=256) -> (vi reference=w741:refnum<vi>, error out=w736:errorcluster)  [unwired: 3 in]
                n424 = call-by-ref "Start Asynchronous Call"(reference=w741, error in=w736) -> ()  [unwired: 12 in, 2 out]
              }
              frame "PMT_SETTINGS" {
                n425 = vi-ref "CameraSettingsMenu.vi"() -> (w744:refnum<vi>)
                n426 = call <vilib>:"Application Directory.vi"() -> ("Application Directory"=w746:path)
                n427 = Build Path(base path=w746, name or relative path="VIs\\Camera\\CameraSettingsMenu.vi") -> (appended path=w743:path)
                n428 = Open VI Reference(type specifier VI Refnum (for type only)=w744, vi path=w743, options=256) -> (vi reference=w747:refnum<vi>)  [unwired: 3 in, 1 out]
                n429 = call-by-ref "Start Asynchronous Call"(reference=w747) -> ()  [unwired: 13 in, 2 out]
              }
              frame "STOP_CAMERA", "STOP_PMT" {
                n430 = global read "GlobalImagingStatus.vi" "ImagingStatus"() -> (w749:T27)
                n431 = case shown="\"Camera\"" w749 {
                  frame "PMT", Default {
                    n432 = Current VI's Menubar() -> (w753:refnum<k9>)
                    n433 = Set Menu Item Info(7:"RUN_CAMERA" ("item tag"), 9:TRUE ("enabled"), 11:w753) -> (3:w751:refnum<k9>)  [unwired: 4 in, 1 out]
                    n434 = Set Menu Item Info(7:"STOP_PMT" ("item tag"), 9:FALSE ("enabled"), 11:w753) -> (3:w752:refnum<k9>)  [unwired: 4 in, 1 out]
                    n435 = Set Menu Item Info(7:"PMT_LARGE_VIEW" ("item tag"), 9:FALSE ("enabled"), 11:w752) -> ()  [unwired: 4 in, 2 out]
                    n436 = Set Menu Item Info(7:"RUN_PMT" ("item tag"), 9:TRUE ("enabled"), 11:w751) -> ()  [unwired: 4 in, 2 out]
                    n437 = global write "GlobalImagingStatus.vi" "ImagingStatus"(ImagingStatusControl."Idle" ("ImagingStatus")) -> ()
                  }
                  frame "Camera" {
                    n438 = Current VI's Menubar() -> (w771:refnum<k9>)
                    n439 = flat-sequence {
                      frame #0 {
                        n440 = global write "GlobalImagingStatus.vi" "ImagingStatus"(ImagingStatusControl."Idle" ("ImagingStatus")) -> ()
                      }
                      frame #1 {
                        n441 = call "CameraCtrl.vi"("Enum"=enum16{"Start", "Stop", "Acquire", "Update"}."Start") -> ()  [unwired: 8 in, 3 out]
                      }
                    }
                    n442 = Set Menu Item Info(7:"RUN_PMT" ("item tag"), 9:TRUE ("enabled"), 11:w771) -> (0:w763:errorcluster, 3:w765:refnum<k9>)  [unwired: 4 in]
                    n443 = Set Menu Item Info(7:"STOP_CAMERA" ("item tag"), 8:w763, 9:FALSE ("enabled"), 11:w765) -> (0:w762:errorcluster, 3:w764:refnum<k9>)  [unwired: 3 in]
                    n444 = Set Menu Item Info(7:"RUN_CAMERA" ("item tag"), 8:w762, 9:TRUE ("enabled"), 11:w764) -> ()  [unwired: 3 in, 2 out]
                  }
                }
              }
              frame "RUN_CAMERA" {
                n445 = flat-sequence {
                  frame #0 {
                    n446 = global read "GlobalCamSettings.vi" "Camera Settings"() -> (w787:T38)
                    n447 = call "CameraCtrl.vi"("Enum"=enum16{"Start", "Stop", "Acquire", "Update"}."Start") -> ("error constant 2"=w788:errorcluster)  [unwired: 8 in, 2 out]
                    n448 = call "CameraCtrl.vi"("error constant"=w788, "Camera Settings"=w787, "Enum"=enum16{"Start", "Stop", "Acquire", "Update"}."Update") -> ()  [unwired: 6 in, 3 out]
                  }
                  frame #1 {
                    n449 = global write "GlobalImagingStatus.vi" "ImagingStatus"(ImagingStatusControl."Camera" ("ImagingStatus")) -> ()
                  }
                }
                n450 = Current VI's Menubar() -> (w782:refnum<k9>)
                n451 = Set Menu Item Info(7:"RUN_PMT" ("item tag"), 9:FALSE ("enabled"), 11:w782) -> (3:w779:refnum<k9>)  [unwired: 4 in, 1 out]
                n452 = Set Menu Item Info(7:"STOP_PMT" ("item tag"), 9:FALSE ("enabled"), 11:w779) -> (3:w778:refnum<k9>)  [unwired: 4 in, 1 out]
                n453 = Set Menu Item Info(7:"RUN_CAMERA" ("item tag"), 9:FALSE ("enabled"), 11:w778) -> (3:w775:refnum<k9>)  [unwired: 4 in, 1 out]
                n454 = Set Menu Item Info(7:"STOP_CAMERA" ("item tag"), 9:TRUE ("enabled"), 11:w775) -> ()  [unwired: 4 in, 2 out]
              }
              frame "RUN_PMT" {
                n455 = Current VI's Menubar() -> (w798:refnum<k9>)
                n456 = Set Menu Item Info(7:"RUN_CAMERA" ("item tag"), 9:FALSE ("enabled"), 11:w798) -> (3:w795:refnum<k9>)  [unwired: 4 in, 1 out]
                n457 = global write "GlobalImagingStatus.vi" "ImagingStatus"(ImagingStatusControl."PMT" ("ImagingStatus")) -> ()
                n458 = Set Menu Item Info(7:"STOP_CAMERA" ("item tag"), 9:FALSE ("enabled"), 11:w795) -> (3:w796:refnum<k9>)  [unwired: 4 in, 1 out]
                n459 = Set Menu Item Info(7:"RUN_PMT" ("item tag"), 9:FALSE ("enabled"), 11:w796) -> (3:w797:refnum<k9>)  [unwired: 4 in, 1 out]
                n460 = Set Menu Item Info(7:"STOP_PMT" ("item tag"), 9:TRUE ("enabled"), 11:w797) -> (3:w792:refnum<k9>)  [unwired: 4 in, 1 out]
                n461 = Set Menu Item Info(7:"PMT_LARGE_VIEW" ("item tag"), 9:TRUE ("enabled"), 11:w792) -> ()  [unwired: 4 in, 2 out]
              }
              frame "SB_COOLING_OPTIONS" {
                n462 = vi-ref "SBCoolingOperationWindow.vi"() -> (w809:refnum<vi>)
                n463 = call <vilib>:"Application Directory.vi"() -> ("Application Directory"=w813:path)
                n464 = Build Path(base path=w813, name or relative path="VIs\\PostProc\\SBCoolingOperationWindow.vi") -> (appended path=w811:path)
                n465 = Open VI Reference(type specifier VI Refnum (for type only)=w809, vi path=w811, options=256) -> (vi reference=w808:refnum<vi>, error out=w810:errorcluster)  [unwired: 3 in]
                n466 = call-by-ref "Start Asynchronous Call"(reference=w808, error in=w810) -> ()  [unwired: 12 in, 2 out]
              }
            }
          }
          event "TreeFolderPath": Value Change {
            n467 = event-data() -> ("NewVal"=w816:path)  [unwired: 1 in]
            n468 = control-ref of="DataTree"() -> (w815:refnum<vi>)
            n469 = call "ExplorerTreeUpdate.vi"("Tree ref"=w815, "Folder Path"=w816) -> ()  [unwired: 10 in]
          }
          event "Process Statedet": Value Change {
            n470 = event-data() -> ()  [unwired: 1 in, 1 out]
            n471 = local read "Compiler Settings"() -> (w817:T18)
            n472 = local read "DataTree"() -> (w818:string)
            n473 = call "RunPythonStateDet.vi"("filepath"=w818, "Compiler Settings"=w817) -> ("standard error"=w820:string, "standard output"=w819:string)  [unwired: 7 in, 1 out]
            n474 = local write "Console Out"(w819) -> ()
            n475 = local write "Python Error Out"(w820) -> ()
          }
          event "LoadPulseSeq": Value Change {
            n476 = event-data() -> ()  [unwired: 1 in, 6 out]
            n477 = local read "DataTree"() -> (w830:string)
            n478 = Build Path(name or relative path=w830) -> (appended path=w829:path)  [unwired: 1 in]
            n479 = call "CompileReadHDF5PulseSeq.vi"("path"=w829) -> ("parameter_config"=w821:string, "pulse_seq_out"=w827:string)  [unwired: 9 in]
            n480 = call "CompileParsePulseSeq.vi"("PulseSeqIn"=w827) -> ("RFPulseList"=w828:string, "PulseList"=w826:T36[])  [unwired: 7 in, 2 out]
            n481 = call "CompileParseMWPulse.vi"("Pulse List In"=w826) -> ("Pulse seq out"=w824:T37)
            n482 = call "CompileParseRFPulse.vi"("String"=w828) -> ("Array"=w825:variant[])  [unwired: 1 in]
            n483 = local write "pulseseq parameter config"(w821) -> ()
            n484 = call "CompileParseAWGPulse.vi"("RF Array"=w825) -> ("MWout"=w823:T9[], "RFout"=w822:T9[])
            n485 = local write "MainPulseSeq"(w824) -> ()
            n486 = local write "MW sequence array"(w823) -> ()
            n487 = local write "RF sequence array"(w822) -> ()
          }
          event "DisplayImage": Value Change {
            n488 = event-data() -> ()  [unwired: 1 in, 1 out]
            n489 = control-ref of="PostProcImg"() -> (w831:refnum<vi>)
            n490 = local read "DataTree"() -> (w833:string)
            n491 = String To Path(string=w833) -> (path=w834:path)
            n492 = call "UpdateMathsPic.vi"("Path"=w834, "ref pic in"=w831) -> ("pic out"=w832:picture)  [unwired: 9 in]
            n493 = local write "PostProcImg"(w832) -> ()
          }
          event "Find Probabilites": Value Change {
            n494 = event-data() -> ()  [unwired: 1 in, 1 out]
            n495 = stacked-sequence {
              frame #0 {
                n496 = local read "Compiler Settings"() -> (w836:T18)
                n497 = local read "NumIonsProcProbs"() -> (w835:bool)
                n498 = control-ref of="Prob graph"() -> (w838:refnum<vi>)
                n499 = local read "DataTree"() -> (w837:string)
                n500 = call "RunPythonFindProbs.vi"("NumIons"=w835, "Prob graph ref"=w838, "Compiler Settings"=w836, "filepath"=w837) -> ("standard error"=w840:string, "standard output"=w839:string)  [unwired: 6 in]
                n501 = local write "Python Error Out"(w840) -> ()
                n502 = local write "Console Out"(w839) -> ()
              }
              frame #1 {
                n503 = local read "TreeFolderPath"() -> (w841:path)
                n504 = control-ref of="DataTree"() -> (w842:refnum<vi>)
                n505 = call "ExplorerTreeUpdate.vi"("Tree ref"=w842, "Folder Path"=w841) -> ()  [unwired: 10 in]
              }
            }
          }
          event "Analyze Probs": Value Change {
            n506 = event-data() -> ()  [unwired: 1 in, 1 out]
            n507 = stacked-sequence {
              frame #0 {
                n508 = local read "Compiler Settings"() -> (w845:T18)
                n509 = local read "DataTree"() -> (w846:string)
                n510 = call "RunPythonProcessData.vi"("Compiler Settings"=w845, "filepath"=w846) -> ("standard error"=w843:string, "standard output"=w844:string)  [unwired: 8 in]
                n511 = local write "Python Error Out"(w843) -> ()
                n512 = local write "Console Out"(w844) -> ()
              }
              frame #1 {
                n513 = local read "TreeFolderPath"() -> (w847:path)
                n514 = control-ref of="DataTree"() -> (w848:refnum<vi>)
                n515 = call "ExplorerTreeUpdate.vi"("Tree ref"=w848, "Folder Path"=w847) -> ()  [unwired: 10 in]
              }
            }
          }
          event Value Change {
            w851 = cluster{"min":i16, "max":i16} {"min"=0, "max"=0} ("SlideBounds")
            n516 = event-data() -> ("NewVal.Left :"=w855:dbl, "NewVal.Right :"=w854:dbl, "NewVal.Bottom :"=w850:dbl, "NewVal.Top :"=w849:dbl)  [unwired: 1 in]
            n517 = Bundle By Name(cluster=w851, "min"=w855, "max"=w854) -> (w856:cluster{"min":i16, "max":i16})
            n518 = Bundle By Name(cluster=w851, "min"=w850, "max"=w849) -> (w852:cluster{"min":i16, "max":i16})
            n519 = control-ref of="CamXSlide"() -> (w857:refnum<vi>)
            n520 = property class="XHorizontalSlide (strict)"(reference=w857, "Property"=w856) -> ()  [unwired: 1 in, 2 out]
            n521 = control-ref of="CamYSlider"() -> (w853:refnum<vi>)
            n522 = property class="XVerticalSlide (strict)"(reference=w853, "Property"=w852) -> ()  [unwired: 1 in, 2 out]
          }
          event "CamXSlide", "CamYSlider": Value Change {
            n523 = event-data() -> ()  [unwired: 1 in, 1 out]
            n524 = control-ref of="CamXSlide"() -> (w860:refnum<vi>)
            n525 = control-ref of="Big Camera"() -> (w858:refnum<vi>)
            n526 = control-ref of="CamYSlider"() -> (w859:refnum<vi>)
            n527 = call "CamUpdateSelectorRect.vi"("large cam ref"=w858, "XVerticalSlide"=w859, "XHorizontalSlide"=w860) -> ()  [unwired: 9 in]
          }
          event "AverageCamera": Value Change {
            n528 = event-data() -> ()  [unwired: 1 in, 6 out]
            n529 = local read "Compiler Settings"() -> (w864:T18)
            n530 = local write "AverageCamera"(FALSE ("AverageCamera")) -> ()
            n531 = call "RunPythonCameraAverage.vi"("Compiler Settings"=w864) -> ("standard error"=w862:string, "standard output"=w863:string)  [unwired: 9 in]
            n532 = local write "Console Out"(w863) -> ()
            n533 = local write "Python Error Out"(w862) -> ()
          }
        }
      }
      n534 = while {
        stop <- w295 stop-if-true
        # "Experiment Controller"
        n535 = event shown="[0] Timeout" {
          selector: _ -> [_ _ _ _ _ _ _ _ _ _ _ _ _ _ _ _ _ _ _]
          dyn-events: _ -> [_ _ _ _ _ _ _ _ _ _ _ _ _ _ _ _ _ _ _]
          timeout: 50 -> [_ _ _ _ _ _ _ _ _ _ _ _ _ _ _ _ _ _ _]
          event Timeout {
            n536 = event-data() -> ()  [unwired: 1 in, 3 out]
            n537 = local write "RunExp"(FALSE ("RunMain")) -> ()
            n538 = stacked-sequence {
              frame #0 {
                n539 = disable-structure shown="Disabled" {
                  frame Disabled {
                    n540 = call "FPGA_ReadAI.vi"() -> ()  [unwired: 11 in, 1 out]
                    n541 = local read item#-1() -> ()  [unwired: 1 in]
                  }
                  frame Enabled {
                  }
                }
              }
              frame #1 {
                n542 = global read "GlobalImagingStatus.vi" "ImagingStatus"() -> (w299:T27)
                n543 = case shown="\"Idle\", Default" w299 {
                  frame "PMT" {
                    n544 = control-ref of="PMT chart"() -> (w300:refnum<vi>)
                    n545 = local read "queue out"() -> (w301:refnum<queue>)
                    n546 = disable-structure shown="PMT_SIMULATED==FALSE" {
                      disable-tunnel: enum16{"READ", "WRITE"}."READ" ("Enum") -> [_ w307]
                      disable-tunnel: [_ w306] -> _
                      disable-tunnel: w301 -> [w303 w305]
                      disable-tunnel: w300 -> [w304 _]
                      frame condition #0 (active) {
                        n547 = call "PMTreadgraph.vi"("queue in"=w303, "PMT chart"=w304) -> ()  [unwired: 9 in, 1 out]
                      }
                      frame condition #1 {
                        n548 = call "PMTreadwriteDEBUG.vi"("Enum"=w307, "queue out"=w305) -> ("Count Chart"=w306:T39)  [unwired: 8 in, 1 out]
                      }
                    }
                  }
                  frame "Idle", Default {
                  }
                }
              }
              frame #2 {
                # "Photodiode fluorescence"
                n549 = disable-structure shown="Enabled" {
                  frame Enabled {
                    n550 = local read "AOMsetting"() -> (w310:T23)
                    n551 = call "AOMReadWrite.vi"("Enum"=enum16{"READ", "WRITE"}."READ") -> ("AOM signal"=w309:fxp<+/-,19,14>, "Photodiode"=w311:dbl)  [unwired: 8 in, 1 out]
                    n552 = in-place {
                      in-place-border: w309 -> [w313]
                      n553 = in-place-cluster #6(w310) -> ()  [unwired: 1 out]
                      n554 = in-place-cluster #6("AOMout"=w313) -> (w308:T23)
                    }
                    n555 = local write "Photodiode"(w311) -> ()
                    n556 = local write "AOMsetting"(w308) -> ()
                  }
                  frame Disabled {
                    n557 = call "AOMdebug.vi"() -> ()  [unwired: 12 in]
                  }
                }
              }
              frame #3 {
                # "MW power"
                n558 = local read "Connection Status"() -> (w315:T17)
                n559 = Unbundle By Name(w315) -> ("rsnrpz"=w314:bool)
                n560 = case shown="True" w314 {
                  frame False {
                  }
                  frame True {
                    n561 = local read "rsnrpz VISA session"() -> (w323:refnum<visa-resource-name>)
                    n562 = control-ref of="RSNPRZsettings"() -> (w318:refnum<vi>)
                    n563 = call "RSNRPZctrl.vi"("VISA session in"=w323, "action"=enum16{"close", "update", "read", "init"}."read") -> ("Measurement"=w319:dbl, "error out"=w322:errorcluster)  [unwired: 10 in, 2 out]
                    n564 = control-ref of="RSNPRZgraph"() -> (w320:refnum<vi>)
                    n565 = control-ref of="Rolling average :"() -> (w316:refnum<vi>)
                    n566 = call "RSNRPZshowMeasurement.vi"("error in (no error)"=w322, "Rolling average : 3"=w316, "Measurement"=w319, "RSNPRZgraph 2"=w320) -> ("power out"=w317:dbl)  [unwired: 6 in, 1 out]
                    n567 = call "RSNRPZpid.vi"("RSNPRZsettings"=w318, "av power in"=w317) -> ()  [unwired: 10 in]
                  }
                }
              }
            }
            n568 = global write "exp_status.vi" "Status"("0" ("Status")) -> ()
          }
          event Value Change {
            w329 = cluster{"min":i16, "max":i16} {"min"=0, "max"=0} ("SlideBounds")
            n569 = event-data() -> ("NewVal"=w331:T11)  [unwired: 1 in]
            n570 = Unbundle By Name(w331) -> ("Top :"=w327:dbl, "Bottom :"=w326:dbl, "Left :"=w325:dbl, "Right :"=w324:dbl)
            n571 = Bundle By Name(cluster=w329, "min"=w326, "max"=w327) -> (w330:cluster{"min":i16, "max":i16})
            n572 = Bundle By Name(cluster=w329, "min"=w325, "max"=w324) -> (w328:cluster{"min":i16, "max":i16})
            n573 = property on="CamYSlider" class="XVerticalSlide (strict)"("Property"=w330) -> ()  [unwired: 2 in, 2 out]
            n574 = property on="CamXSlide" class="XHorizontalSlide (strict)"("Property"=w328) -> ()  [unwired: 2 in, 2 out]
          }
          event Menu Selection (User) {
            n575 = event-data() -> ("ItemTag"=w332:string)  [unwired: 1 in]
            n576 = case shown="\"PMT_LARGE_VIEW\"" w332 {
              frame "False", Default {
              }
              frame "PMT_LARGE_VIEW" {
                n577 = disable-structure shown="Enabled" {
                  frame Enabled {
                    n578 = call <vilib>:"Application Directory.vi"() -> ("Application Directory"=w343:path)
                    n579 = local read "queue out"() -> (w337:refnum<queue>)
                    n580 = Build Path(base path=w343, name or relative path="VIs\\PMT\\PMTlargeView.vi") -> (appended path=w341:path)
                    n581 = Open VI Reference(type specifier VI Refnum (for type only)=refnum<vi> refnum, vi path=w341, options=128) -> (vi reference=w339:refnum<vi>, error out=w338:errorcluster)  [unwired: 3 in]
                    n582 = call-by-ref "Start Asynchronous Call"(reference=w339, error in=w338, "queue out"=w337) -> (reference out=w336:refnum<vi>, error out=w335:errorcluster)  [unwired: 11 in]
                    n583 = Close Reference(reference=w336, error in (no error)=w335) -> ()  [unwired: 1 out]
                  }
                  frame Disabled {
                  }
                }
                n584 = global read "GlobalImagingStatus.vi" "ImagingStatus"() -> (w333:T27)
                n585 = case shown="\"PMT\"" w333 {
                  selector: w333 -> [w345 _]
                  tunnel: [w345 ImagingStatusControl."PMT_large" ("ImagingStatus")] -> w334
                  frame "Idle", Default {
                  }
                  frame "PMT" {
                  }
                }
                n586 = global write "GlobalImagingStatus.vi" "ImagingStatus"(w334) -> ()
              }
            }
          }
          event "AOMsetting": Value Change {
            n587 = event-data() -> ("NewVal"=w347:T23)  [unwired: 1 in]
            n588 = disable-structure shown="FPGA_ENABLED==TRUE" {
              disable-tunnel: w347 -> [w348 _]
              frame condition #0 (active) {
                n589 = call "AOMReadWrite.vi"("Enum"=enum16{"READ", "WRITE"}."WRITE", "XAOMsetting"=w348) -> ()  [unwired: 7 in, 3 out]
              }
              frame condition #1 {
              }
            }
          }
          event Value Change {
            n590 = event-data() -> ("NewVal"=w350:dbl)  [unwired: 1 in]
            n591 = call "RecrystalliseTCPcomm.vi"("DC voltage in"=w350) -> ()  [unwired: 10 in, 1 out]
          }
          event Value Change {
            n592 = event-data() -> ("NewVal"=w351:dbl)  [unwired: 1 in]
            n593 = In Range and Coerce(upper limit=3000.0, x=w351, lower limit=0.0) -> (coerced(x)=w354:dbl)  [unwired: 1 out]
            n594 = call "AuxSetCurrent.vi"("Enabled?"=TRUE, "Function select"=enum16{"Init", "Set", "Close"}."Set", "current /mA"=w354) -> ()  [unwired: 6 in, 3 out]
          }
          event "Main/Meta": Value Change {
            n595 = event-data() -> ("NewVal"=w357:bool)  [unwired: 1 in]
            n596 = case shown="True" w357 {
              tunnel: w357 -> [w363 w371]
              frame False {
                n597 = property on="ExperimentTab" class="TabCtl (strict)"() -> ("Pages"=w362:refnum<vi>[])  [unwired: 2 in, 2 out]
                n598 = Index Array(array=w362, index=1) -> (element=w360:refnum<vi>)
                n599 = global read "GlobalExp.vi" "GlobalExp"() -> (w364:T31)
                n600 = property class="Page"(reference=w360, "PageEnb"=T30."Page Disabled & Grayed" ("Page Enabled State")) -> ()  [unwired: 1 in, 2 out]
                n601 = Bundle By Name(cluster=w364, "Main/Meta"=w363) -> (w365:T31)
                n602 = global write "GlobalExp.vi" "GlobalExp"(w365) -> ()
                n603 = property on="MetaPush" class="Bool (strict)"("DisabledEnum"=T28."Disabled and Grayed Out" ("Disabled")) -> ()  [unwired: 2 in, 2 out]
              }
              frame True {
                n604 = property on="ExperimentTab" class="TabCtl (strict)"() -> ("Pages"=w367:refnum<vi>[])  [unwired: 2 in, 2 out]
                n605 = flat-sequence {
                  tunnel: w371 -> [w373]
                  frame #0 {
                    n606 = local read "Compiler Settings"() -> (w372:T18)
                    n607 = call "MetaLaunchPythonServer.vi"("Compiler Settings"=w372) -> ()  [unwired: 11 in]
                  }
                  frame #1 {
                    n608 = global read "GlobalExp.vi" "GlobalExp"() -> (w374:T31)
                    n609 = Bundle By Name(cluster=w374, "Main/Meta"=w373) -> (w375:T31)
                    n610 = global write "GlobalExp.vi" "GlobalExp"(w375) -> ()
                  }
                }
                n611 = Index Array(array=w367, index=1) -> (element=w369:refnum<vi>)
                n612 = property on="MetaPush" class="Bool (strict)"("DisabledEnum"=T28."Enabled" ("Disabled")) -> ()  [unwired: 2 in, 2 out]
                n613 = property class="Page"(reference=w369, "PageEnb"=T30."Page Enabled" ("Page Enabled State")) -> ()  [unwired: 1 in, 2 out]
              }
            }
          }
          event "RunExp": Value Change {
            n614 = event-data() -> ()  [unwired: 1 in, 6 out]
            n615 = global read "GlobalImagingStatus.vi" "ImagingStatus"() -> (w376:T27)
            n616 = local read "Main/Meta"() -> (w377:bool)
            n617 = stacked-sequence {
              tunnel: w377 -> [_ w398 _ _ _ _]
              tunnel: w376 -> [_ _ _ w449 w457 _]
              frame #0 {
                w379 = T28."Disabled and Grayed Out" ("Disabled")
                # "Disable menu items for PMT/Cam, AOM ctrl"
                n618 = control-ref of="AOMsetting"() -> (w380:refnum<vi>)
                n619 = property class="XAOMsetting (strict)"(reference=w380, "DisabledEnum"=w379) -> ()  [unwired: 1 in, 2 out]
                n620 = Current VI's Menubar() -> (w385:refnum<k9>)
                n621 = Set Menu Item Info(7:"RUN_PMT" ("item tag"), 9:FALSE ("enabled"), 11:w385) -> ()  [unwired: 4 in, 2 out]
                n622 = Set Menu Item Info(7:"RUN_CAMERA" ("item tag"), 9:FALSE ("enabled"), 11:w385) -> ()  [unwired: 4 in, 2 out]
                n623 = control-ref of="PMT chart"() -> (w384:refnum<vi>)
                n624 = property class="WFChart (strict)"(reference=w384, "DisabledEnum"=w379) -> ()  [unwired: 1 in, 2 out]
                n625 = global write "DataLock.vi" "Lock"(FALSE ("Lock")) -> ()
                n626 = Set Menu Item Info(7:"STOP_PMT" ("item tag"), 9:FALSE ("enabled"), 11:w385) -> ()  [unwired: 4 in, 2 out]
                n627 = Set Menu Item Info(7:"STOP_CAMERA" ("item tag"), 9:FALSE ("enabled"), 11:w385) -> ()  [unwired: 4 in, 2 out]
                n628 = global write "GraphsQueue.vi" "GraphQueue"(i16 0 ("Numeric")) -> ()
                n629 = Set Menu Item Info(7:"RUN_CAMERA" ("item tag"), 9:FALSE ("enabled"), 11:w385) -> ()  [unwired: 4 in, 2 out]
                n630 = control-ref of="Small Camera"() -> (w383:refnum<vi>)
                n631 = property class="IntGraph (strict)"(reference=w383, "DisabledEnum"=w379) -> ()  [unwired: 1 in, 2 out]
                n632 = Set Menu Item Info(7:"RUN_PMT" ("item tag"), 9:FALSE ("enabled"), 11:w385) -> ()  [unwired: 4 in, 2 out]
                n633 = global write "GlobalImagingStatus.vi" "ImagingStatus"(ImagingStatusControl."Idle" ("ImagingStatus")) -> ()
                n634 = call "ResetQueue.vi"() -> ()  [unwired: 11 in, 1 out]
              }
              frame #1 {
                # "Main controller"
                n635 = case shown="True" w398 {
                  frame False {
                    # "Main"
                    n636 = local read "Compiler Settings"() -> (w404:T18)
                    n637 = local read "Param Cfg Path"() -> (w401:path)
                    n638 = local read "ion coords"() -> (w399:T11)
                    n639 = local read "File Paths"() -> (w403:T19)
                    n640 = call "ContMainInit.vi"("ion coords"=w399, "configuration file path"=w401, "File Paths"=w403, "Compiler Settings"=w404) -> ("kinetic img size"=w400:cluster{"xpixels":i32, "ypixels":i32}, "steps"=w402:dbl)  [unwired: 6 in]
                    n641 = Not Equal To 0?(x=w402) -> (x != 0?=w405:bool)
                    n642 = case shown="True" w405 {
                      tunnel: w402 -> [_ w417]
                      tunnel: w400 -> [_ w416]
                      frame False {
                      }
                      frame True {
                        n643 = control-ref of="ControllerSettings"() -> (w407:refnum<vi>)
                        n644 = control-ref of="Mean graph"() -> (w421:refnum<vi>)
                        n645 = control-ref of="Raw graph"() -> (w422:refnum<vi>)
                        n646 = control-ref of="Proc. graph"() -> (w420:refnum<vi>)
                        n647 = local read "Compiler Settings"() -> (w419:T18)
                        n648 = local read "File Paths"() -> (w418:T19)
                        n649 = control-ref of="steps slider"() -> (w415:refnum<vi>)
                        n650 = control-ref of="runs slider"() -> (w414:refnum<vi>)
                        n651 = control-ref of="CompCoilSettings"() -> (w408:refnum<vi>)
                        n652 = Bundle("steps slider"=w415, "runs slider"=w414) -> (w413:T40)  [unwired: 1 in]
                        n653 = control-ref of="Aux graph"() -> (w410:refnum<vi>)
                        n654 = control-ref of="PowerStableSettings"() -> (w406:refnum<vi>)
                        n655 = control-ref of="FluoSettings"() -> (w412:refnum<vi>)
                        n656 = call "GraphsUpdateMain.vi"("raw graph ref"=w422, "File Paths"=w418, "Compiler Settings"=w419, "mean graph ref"=w421, "proc graph ref"=w420, "ControllerSettingsRef"=w407) -> ()  [unwired: 9 in, 1 out]
                        n657 = control-ref of="AOMsetting"() -> (w409:refnum<vi>)
                        n658 = Bundle("CompCoilSettings"=w408, "FluoSettings"=w412, "AOMsetting"=w409, "PowerStableSettings"=w406) -> (w411:T41)  [unwired: 1 in]
                        n659 = call "ContMain.vi"("CtrlRefsin"=w411, "Aux chart ref in"=w410, "steps"=w417, "slider refs in"=w413, "kinetic img size"=w416, "File Paths"=w418, "Compiler Settings"=w419, "ControllerSettingsRef"=w407) -> ()  [unwired: 4 in]
                      }
                    }
                  }
                  frame True {
                    # "Meta"
                    n660 = control-ref of="ControllerSettings"() -> (w424:refnum<vi>)
                    n661 = control-ref of="Raw graph"() -> (w429:refnum<vi>)
                    n662 = control-ref of="Mean graph"() -> (w428:refnum<vi>)
                    n663 = control-ref of="Proc. graph"() -> (w427:refnum<vi>)
                    n664 = local read "Compiler Settings"() -> (w425:T18)
                    n665 = local read "File Paths"() -> (w426:T19)
                    n666 = local write "RunExp"(FALSE ("RunExp")) -> ()
                    n667 = control-ref of="FluoSettings"() -> (w432:refnum<vi>)
                    n668 = call "GraphsUpdateMeta.vi"("raw graph ref"=w429, "File Paths"=w426, "Compiler Settings"=w425, "mean graph ref"=w428, "proc graph ref"=w427, "ControllerSettingsRef"=w424) -> ()  [unwired: 9 in, 1 out]
                    n669 = control-ref of="StepsSlider"() -> (w436:refnum<vi>)
                    n670 = control-ref of="CompCoilSettings"() -> (w433:refnum<vi>)
                    n671 = control-ref of="runs slider"() -> (w437:refnum<vi>)
                    n672 = control-ref of="AOMsetting"() -> (w431:refnum<vi>)
                    n673 = control-ref of="PowerStableSettings"() -> (w423:refnum<vi>)
                    n674 = control-ref of="Aux graph"() -> (w434:refnum<vi>)
                    n675 = Bundle("StepsSlider"=w436, "runs slider"=w437) -> (w435:T42)  [unwired: 1 in]
                    n676 = Bundle("CompCoilSettings"=w433, "FluoSettings"=w432, "AOMsetting"=w431, "PowerStableSettings"=w423) -> (w430:T41)  [unwired: 1 in]
                    n677 = call "ContMeta.vi"("Aux graph ref"=w434, "CtrlRefsin"=w430, "slider refs in"=w435, "File Paths"=w426, "Compiler Settings"=w425, "ControllerSettingsRef"=w424) -> ()  [unwired: 6 in]
                  }
                }
              }
              frame #2 {
                w439 = FALSE
                n678 = local read "Pause/Stop"() -> (w440:cluster{"Exp Stop":bool, "Pause":bool})
                n679 = Bundle By Name(cluster=w440, "Exp Stop"=FALSE) -> (w441:cluster{"Exp Stop":bool, "Pause":bool})
                n680 = property on="RunExp" class="Bool (strict)"("DisabledEnum"=T28."Disabled and Grayed Out" ("Disabled")) -> (error out=w447:errorcluster)  [unwired: 2 in, 1 out]
                n681 = local write "Pause/Stop"(w441) -> ()
                n682 = global read "GlobalExp.vi" "GlobalExp"() -> (w443:T31)
                n683 = property on="RunExp" class="Bool (strict)"(error in=w447, "DisabledEnum"=T28."Enabled" ("Disabled")) -> ()  [unwired: 1 in, 2 out]
                n684 = Bundle By Name(cluster=w443, "MetaExpOver"=w439, "Stop"=w439, "ExpStatus"=T29."Idle") -> (w444:T31)
                n685 = global write "GlobalExp.vi" "GlobalExp"(w444) -> ()
              }
              frame #3 {
                # "Reset camera"
                n686 = Equal?(x=w449, y=ImagingStatusControl."Camera") -> (x = y?=w451:bool)
                n687 = case shown="True" w451 {
                  frame False {
                  }
                  frame True {
                    n688 = global read "GlobalCamSettings.vi" "Camera Settings"() -> (w454:T38)
                    n689 = call "CameraCtrl.vi"("error constant"=errorcluster {"status"=FALSE, "code"=0, "source"=""}, "Enum"=enum16{"Start", "Stop", "Acquire", "Update"}."Start") -> ("error constant 2"=w455:errorcluster)  [unwired: 7 in, 2 out]
                    n690 = call "CameraCtrl.vi"("error constant"=w455, "Camera Settings"=w454, "Enum"=enum16{"Start", "Stop", "Acquire", "Update"}."Update") -> ()  [unwired: 6 in, 3 out]
                  }
                }
              }
              frame #4 {
                w461 = T28."Enabled" ("Disabled")
                # "Reenable menu items"
                n691 = control-ref of="AOMsetting"() -> (w458:refnum<vi>)
                n692 = property class="XAOMsetting (strict)"(reference=w458, "DisabledEnum"=w461) -> ()  [unwired: 1 in, 2 out]
                n693 = global write "GlobalImagingStatus.vi" "ImagingStatus"(w457) -> ()
                n694 = Current VI's Menubar() -> (w462:refnum<k9>)
                n695 = control-ref of="PMT chart"() -> (w460:refnum<vi>)
                n696 = property class="WFChart (strict)"(reference=w460, "DisabledEnum"=w461) -> ()  [unwired: 1 in, 2 out]
                n697 = Set Menu Item Info(7:"RUN_PMT" ("item tag"), 9:TRUE ("enabled"), 11:w462) -> ()  [unwired: 4 in, 2 out]
                n698 = Set Menu Item Info(7:"RUN_CAMERA" ("item tag"), 9:TRUE ("enabled"), 11:w462) -> ()  [unwired: 4 in, 2 out]
                n699 = Set Menu Item Info(7:"STOP_PMT" ("item tag"), 9:TRUE ("enabled"), 11:w462) -> ()  [unwired: 4 in, 2 out]
                n700 = Set Menu Item Info(7:"STOP_CAMERA" ("item tag"), 9:TRUE ("enabled"), 11:w462) -> ()  [unwired: 4 in, 2 out]
                n701 = control-ref of="Small Camera"() -> (w459:refnum<vi>)
                n702 = property class="IntGraph (strict)"(reference=w459, "DisabledEnum"=w461) -> ()  [unwired: 1 in, 2 out]
                n703 = Set Menu Item Info(7:"RUN_CAMERA" ("item tag"), 9:TRUE ("enabled"), 11:w462) -> ()  [unwired: 4 in, 2 out]
                n704 = Set Menu Item Info(7:"RUN_PMT" ("item tag"), 9:TRUE ("enabled"), 11:w462) -> ()  [unwired: 4 in, 2 out]
              }
              frame #5 {
                # "Update post processing image and tree"
                n705 = local read "TreeFolderPath"() -> (w479:path)
                n706 = local read "MathImageCtl"() -> (w480:T5)
                n707 = Unbundle By Name(w480) -> ("Auto update :"=w481:bool)
                n708 = control-ref of="DataTree"() -> (w478:refnum<vi>)
                n709 = call "ExplorerTreeUpdate.vi"("Tree ref"=w478, "Folder Path"=w479) -> ()  [unwired: 10 in]
                n710 = case shown="True" w481 {
                  tunnel: w480 -> [_ w488]
                  frame False {
                  }
                  frame True {
                    n711 = local read "File Paths"() -> (w491:T19)
                    n712 = global read "GlobalExp.vi" "GlobalExp"() -> (w486:T31)
                    n713 = control-ref of="PltPic"() -> (w490:refnum<vi>)
                    n714 = Unbundle By Name(w486) -> ("date"=w485:string, "ExpNum"=w483:dbl)
                    n715 = Format Into String(format string="%03d", w483) -> (resulting string=w484:string)  [unwired: 2 in, 1 out]
                    n716 = Bundle By Name(cluster=w488, "Date:"=w485, "Exp Num:"=w484) -> (w487:T5)
                    n717 = call "UpdateMathsPic.vi"("ref pic in"=w490, "File Paths"=w491, "MathImageCtl"=w487) -> ("pic out"=w489:picture)  [unwired: 8 in]
                    n718 = local write "PltPic"(w489) -> ()
                  }
                }
                n719 = local read "ArbitraryWaveListMW"() -> (w475:dbl[][])
                n720 = call "AWGCompileContinuousWave.vi"("ArbitraryWaveListMW"=w475) -> ("error out"=w476:errorcluster, "array MW and RF"=w477:variant[])  [unwired: 1 in]
                n721 = call "AWGSendPulseArrayContinuous.vi"("error in (no error)"=w476, "AWG pulses array"=w477) -> ()  [unwired: 8 in, 2 out]
              }
            }
          }
          event Value Change {
            n722 = event-data() -> ("NewVal"=w496:dbl)  [unwired: 1 in]
            n723 = local read "Agilient visa"() -> (w494:string)
            n724 = Type Cast(type=refnum<visa-resource-name> "TCPIP0::192.168.1.203::inst0::INSTR" ("VISA resource name"), x=w494) -> (*(type *) &x=w492:refnum<visa-resource-name>)
            n725 = call "AgilientVSGCtrl.vi"("action"=AgilentCtrlEnum."WRITE_POW", "pow write"=w496, "VISA resource name"=w492) -> ()  [unwired: 7 in, 2 out]
          }
          event Value Change {
            n726 = event-data() -> ("NewVal"=w497:bool)  [unwired: 1 in]
            n727 = global read "GlobalExp.vi" "GlobalExp"() -> (w498:T31)
            n728 = Bundle By Name(cluster=w498, "Camera"=w497) -> (w499:T31)
            n729 = global write "GlobalExp.vi" "GlobalExp"(w499) -> ()
          }
          event "DIOcluster": Value Change {
            n730 = event-data() -> ("NewVal"=w501:T14)  [unwired: 1 in]
            n731 = call "FPGAReadWrite.vi"("Enum"=enum16{"WRITE_DIO", "WRITE_AO", "READ_AI"}."WRITE_DIO", "DIOcluster"=w501) -> ()  [unwired: 8 in, 2 out]
          }
          event "DisconnectCamera": Value Change {
            n732 = event-data() -> ("NewVal"=w502:bool)  [unwired: 1 in]
            n733 = global read "GlobalImagingStatus.vi" "ImagingStatus"() -> (w506:T27)
            n734 = Equal?(x=w506, y=ImagingStatusControl."Idle") -> (x = y?=w503:bool)
            n735 = And(x=w502, y=w503) -> (x .and. y?=w504:bool)
            n736 = case shown="True" w504 {
              frame False {
              }
              frame True {
                n737 = call "CameraShutdown.vi"() -> ("error out"=w508:errorcluster)  [unwired: 1 in]
                n738 = local write "DisconnectCamera"(FALSE ("DisconnectCamera")) -> ()
                n739 = case shown="Error" w508 {
                  selector: w508 -> [_ w512]
                  tunnel: ["Shutdown Success" ("Shutdown Status :") w511] -> w507
                  frame No Error {
                  }
                  frame Error {
                    n740 = Unbundle By Name(w512) -> ("source"=w511:string)
                  }
                }
                n741 = local write "Shutdown Status :"(w507) -> ()
              }
            }
          }
          event "camera debug": Value Change {
            n742 = event-data() -> ()  [unwired: 1 in, 6 out]
            n743 = local write "camera debug"(FALSE ("camera debug")) -> ()
            n744 = disable-structure shown="Disabled" {
              frame Disabled {
                n745 = call "CameraKineticDEBUG.vi"() -> ()  [unwired: 12 in]
              }
              frame Enabled {
              }
            }
          }
          event "UpdateAWGGraph": Value Change {
            n746 = event-data() -> ()  [unwired: 1 in, 3 out]
            n747 = local write "UpdateAWGGraph"(FALSE ("UpdateAWGGraph")) -> ()
            n748 = control-ref of="Wave Form preview"() -> (w516:refnum<vi>)
            n749 = local read "ArbitraryWaveListMW"() -> (w514:dbl[][])
            n750 = call "AWGUpdateWaveformViewer.vi"("Wave Form preview ref"=w516, "Item Names"=w514) -> ()  [unwired: 10 in]
          }
          event "SendWaveformToAWG": Value Change {
            n751 = event-data() -> ()  [unwired: 1 in, 6 out]
            n752 = local read "ArbitraryWaveListMW"() -> (w518:dbl[][])
            n753 = control-ref of="Wave Form preview"() -> (w517:refnum<vi>)
            n754 = local write "SendWaveformToAWG"(FALSE ("SendWaveformToAWG")) -> ()
            n755 = call "AWGCompileContinuousWave.vi"("ArbitraryWaveListMW"=w518) -> ("error out"=w520:errorcluster, "array MW and RF"=w521:variant[])  [unwired: 1 in]
            n756 = call "AWGUpdateWaveformViewer.vi"("Wave Form preview ref"=w517, "Item Names"=w518) -> ()  [unwired: 10 in]
            n757 = call "AWGSendPulseArrayContinuous.vi"("error in (no error)"=w520, "AWG pulses array"=w521) -> ("msg out"=w519:string)  [unwired: 8 in, 1 out]
            n758 = local write "AWGContMSG"(w519) -> ()
          }
          event "SaveWaveformsToFile": Value Change {
            n759 = event-data() -> ()  [unwired: 1 in, 6 out]
            n760 = local read "ArbitraryWaveListMW"() -> (w525:dbl[][])
            n761 = local write "SaveWaveformsToFile"(FALSE ("SaveWaveformsToFile")) -> ()
            n762 = call-poly <vilib>:"Write Delimited Spreadsheet.vi"("2D data"=w525) -> ("error out"=w524:errorcluster)  [unwired: 13 in, 1 out]
            n763 = case shown="No Error" w524 {
              frame No Error {
              }
              frame Error {
              }
            }
          }
          event "LoadWaveforms": Value Change {
            n764 = event-data() -> ()  [unwired: 1 in, 6 out]
            n765 = call-poly <vilib>:"Read Delimited Spreadsheet.vi"() -> ("all rows"=w528:dbl[][], "error out"=w527:errorcluster)  [unwired: 10 in, 4 out]
            n766 = local write "LoadWaveforms"(FALSE ("LoadWaveforms")) -> ()
            n767 = case shown="No Error" w527 {
              tunnel: w528 -> [w529 _]
              frame No Error {
                n768 = local write "ArbitraryWaveListMW"(w529) -> ()
              }
              frame Error {
              }
            }
          }
          event Value Change {
            n769 = event-data() -> ("NewVal"=w531:T12)  [unwired: 1 in, 5 out]
            n770 = local read "rsnrpz VISA session"() -> (w532:refnum<visa-resource-name>)
            n771 = call "RSNRPZctrl.vi"("VISA session in"=w532, "RSNPRZsettings"=w531, "action"=enum16{"close", "update", "read", "init"}."update") -> ()  [unwired: 9 in, 4 out]
          }
          event "AO cluster": Value Change {
            n772 = event-data() -> ("NewVal"=w533:T13)  [unwired: 1 in]
            n773 = call "FPGAUpdateAO.vi"("AIO cluster"=w533) -> ()  [unwired: 8 in, 1 out]
          }
        }
        n774 = shared-variable "My Computer\\Global.lvlib\\Stop"() -> (w295:bool)  [unwired: 1 in, 1 out]
      }
    }
    frame #3 {
      # "Shutdown procedure"
      n775 = local read "Running VIs ref"() -> (w871:refnum<vi>[])
      n776 = local read "rsnrpz VISA session"() -> (w866:refnum<visa-resource-name>)
      n777 = disable-structure shown="Disabled" {
        frame Disabled {
          n778 = local read "VISA: Pressure"() -> (w872:refnum<visa-resource-name>)
          n779 = call "DriverVarianXGS-600.vi"("VISA resource name"=w872, "Action"=enum16{"Start", "Read", "Stop"}."Stop") -> ()  [unwired: 1 in, 4 out]
        }
        frame Enabled {
        }
      }
      n780 = call "FPGAref.vi"() -> ("error out"=w869:errorcluster, "FPGA VI Reference Out 2"=w870:refnum<k20>)  [unwired: 6 in]
      n781 = global read "GlobalImagingStatus.vi" "ImagingStatus"() -> (w868:T27)
      n782 = xnode "Close FPGA VI Reference"("FPGA VI Reference In"=w870, "error in"=w869) -> ()  [unwired: 1 out]
      n783 = for {
        tunnel: w871 -> [w877] mode=indexing
        # "Shutdown all running async VIs"
        n784 = invoke class="VI" method="Abort VI"(reference=w877) -> (reference out=w876:refnum<vi>, error out=w875:errorcluster)  [unwired: 2 in, 1 out]
        n785 = Close Reference(reference=w876, error in (no error)=w875) -> ()  [unwired: 1 out]
      }
      n786 = call "RSNRPZctrl.vi"("VISA session in"=w866, "action"=enum16{"close", "update", "read", "init"}."close") -> ()  [unwired: 10 in, 4 out]
      n787 = case shown="\"Camera_large\", \"Camera\"" w868 {
        frame "Camera_large", "Camera" {
          n788 = call "CameraCtrl.vi"("Enum"=enum16{"Start", "Stop", "Acquire", "Update"}."Start") -> ()  [unwired: 8 in, 3 out]
        }
        frame "PMT", Default {
        }
      }
      n789 = call "AuxSetCurrent.vi"("Function select"=enum16{"Init", "Set", "Close"}."Close") -> ()  [unwired: 8 in, 3 out]
    }
  }
  n790 = disable-structure shown="Disabled" {
    frame Disabled {
      n791 = while {
        shift-right: [w885] -> _
        shift-left: _ -> [w884]
        stop <- w881 stop-if-true
        n792 = control-ref of="Small Camera"() -> (w880:refnum<vi>)
        n793 = Get Date/Time String() -> (time string=w878:string)  [unwired: 3 in, 1 out]
        "time string" <- w878
        n794 = Scan From String(format string="%d:%d", input string=w878) -> (output 2=w885:i32)  [unwired: 5 in, 3 out]
        "output 2" <- w885
        n795 = Not Equal?(x=w885, y=w884) -> (x != y?=w883:bool)
        n796 = case shown="True" w883 {
          tunnel: w880 -> [_ w892]
          tunnel: "C:\\Users\\labadmin\\Documents\\Micromotion\\camera_data_2\\" -> [_ w893]
          tunnel: w878 -> [_ w889]
          frame False {
          }
          frame True {
            n797 = property class="IntGraph (strict)"(reference=w892) -> ("Value"=w895:dbl[][])  [unwired: 1 in, 2 out]
            n798 = Search and Replace String(input string=w889, search string=":", replace string="_" ("replace string (\"\")")) -> (result string=w887:string)  [unwired: 5 in, 3 out]
            n799 = Concatenate Strings(w893, w887) -> (w888:string)
            n800 = String To Path(string=w888) -> (path=w894:path)
            n801 = call-poly <vilib>:"Write Delimited Spreadsheet.vi"("file path (dialog if empty)"=w894, "2D data"=w895) -> ()  [unwired: 12 in, 2 out]
          }
        }
        n802 = shared-variable "My Computer\\Global.lvlib\\Stop"() -> (w881:bool)  [unwired: 1 in, 1 out]
        n803 = Wait (ms)(milliseconds to wait=u32 5000) -> ()  [unwired: 1 out]
      }
    }
    frame Enabled {
    }
  }
  n804 = disable-structure shown="Disabled" {
    disable-tunnel: _ -> [w897 _]
    frame Disabled {
      # "Pressure"
      n805 = local read "VISA: Pressure"() -> (w896:refnum<visa-resource-name>)
      n806 = local read "Connection Status"() -> (w901:T17)
      n807 = call "DriverVarianXGS-600.vi"("VISA resource name"=w896, "Action"=enum16{"Start", "Read", "Stop"}."Start", "error in (no error)"=w897) -> ("Pressure connect?"=w900:bool)  [unwired: 3 out]
      n808 = in-place {
        in-place-border: w900 -> [w902]
        n809 = in-place-cluster #7(w901) -> ()  [unwired: 1 out]
        n810 = in-place-cluster #7("Pressure"=w902) -> (w899:T17)
      }
      n811 = local write "Connection Status"(w899) -> ()
    }
    frame Enabled {
    }
  }
